vi "Text control 2 v6.0.vi"() -> ()   [LabVIEW 2016]
panel:
  in  "Tab Control":enum32{"Main", "Other parameters"}(tab)
  out "Line running":i32
  out "Total lines":i32
  out "Path":path=path "C:/users/rlp38/09Apr2009LTtesting/test2.txt"
  out "I vs Vg":cluster{"Y data in":dbl[], "X data in":dbl[]}[](graph)
  out "Is max":dbl format="%.2e"
  out "Id max":dbl format="%.2e"
  out "Ig max":dbl format="%.2e"
  out "Imax vs time":cluster{"Y data in":dbl[], "X data in":dbl[]}[](graph)
  out "Imin vs time":cluster{"Y data in":dbl[], "X data in":dbl[]}[](graph)
  out "I vs Vd":cluster{"Y data in":dbl[], "X data in":dbl[]}[](graph)
  in  "Script":string="#pulsedstressV d 0.03 20 0 0.5 0.0827 5\n#\n#itime m\n#gaterangemode a\n#drainrangemode a\n#pulsed on 0.05 0 0.02\n#transfer d -10 40 1 5 40 35\n#transfer d -10 40 1 5 40 35\n#transfer d -10 40 1 5 40 35\n#output d 0 40 20 0 40 1\n#\n#\n#sample 1 0.008 221 6 0.003\n#samplei 400e-6 200 6 0.002 0.1\n#vsu2pulse -10 4\n#\n#stressV 0.016 0.03 2e-4 0.1e-3 11\n#stressI 220e-7 0.08 15\n#transfer s -1 1 0.5 -0.005 0.005 0.005\n#output s 0 0 0 -0.008 0.008 0.002"
  out "Command running:":string
  out "Serial port data":string
  out "Elapsed Time":dbl caption="Elapsed Time (s)"
  in  "Units (label only)":u16(ring)=1 items=["Seconds", "Minutes", "Hours"]
  in  "Time Offset":dbl caption="Set Start Time (s)"
  in  "Reset":bool
  in  "Auto Reset":bool
  in  "integration time":u32(slide) max=2 step=1 scale=0.0..2.0
  out "Is on":dbl format="%.2e"
  out "Id on":dbl format="%.2e"
  out "Ig on":dbl format="%.2e"
  out "Ion vs time":cluster{"Y data in":dbl[], "X data in":dbl[]}[](graph)
  out "Ioff vs time":cluster{"Y data in":dbl[], "X data in":dbl[]}[](graph)
  out "Ig min":dbl format="%.2e"
  out "Id min":dbl format="%.2e"
  out "Is min":dbl format="%.2e"
  out "Is off":dbl format="%.2e"
  out "Id off":dbl format="%.2e"
  out "Ig off":dbl format="%.2e"
  in  "Integration time (long)":dbl=0.32 min=0.04 max=2.0 step=0.02 format="%.2f"
  in  "Integration time (short)":dbl=0.0019 min=8e-05 max=0.0019 step=8e-05 format="%^.0e"
  in  "Drain: Compliance":dbl=0.001 format="%.8f"
  in  "Gate: Compliance":dbl=0.001 format="%.8f"
  in  "Interrupt run":bool
  in  "Standby":T1
  in  "Full Reset":bool
  in  "SMU4":cluster{"on/off":bool, "Voltage":dbl} {"Voltage" min=-100.0 max=100.0 format="%.2f"}
  in  "Gate Range\nmode":u16(ring) items=["Auto", "Limited", "Fixed"]
  in  "Gate Range":u8(slide)=6 max=11 scale=0.0..11.0
  in  "Source/Drain\nRange mode":u16(ring) items=["Auto", "Limited", "Fixed"]
  in  "Source/Drain Range":u8(slide)=6 max=11 scale=0.0..11.0
  in  "Panel Controls":T2={"Emergency Stop"=refnum, "TransGraph Max"=1e-05, "Text/Graph (text=false)"=TRUE} {"TransGraph Max" format="%.2e"}
  in  "Panel Controls 2":T3={"Emergency Stop"=refnum, "TransGraph Max"=1e-05, "Text/Graph (text=false)"=TRUE, "TransGraph Min"=1e-11} {"TransGraph Min" format="%.2e"; "TransGraph Max" format="%.2e"}
  out "error out":errorcluster
  in  "Delay before read (ms)":u32=1000
  in  "byte count":u32=64
  in  "Serial End Mode for Reads":u16(ring)=2 items=["None", "LastBit", "TermChar"]
  in  "Timeout (ms)":u32=10000
  in  "Enable Termination\nChar (T)":bool=TRUE
  in  "Termination char\n(0xA = '\\n' = LF)\n(0xD = '\\r' = CR)":u8=13 format="%.0x"
  in  "flow control":u16(ring) items=["None"=0, "XON/XOFF"=1, "RTS/CTS"=2, "DTR/DSR"=4]
  in  "stop bits":u16(ring)=10 items=["1.0"=10, "1.5"=15, "2.0"=20]
  in  "parity":u16(ring) items=["None", "Odd", "Even", "Mark", "Space"]
  in  "data bits":u16=8 min=5 max=8 step=1
  in  "VISA resource name":refnum<visa-resource-name>="COM6"
  in  "baud rate":u32=9600
  out "Timings Indicator":T4
  in  "Timings (overwritten by the Front Panel)":T5={"integration time"=0, "Short/Long integration time"=0.00064, "hold time (sec)"=0.0, "delay time (sec)"=0.0, "Step Time (0 disables)"=0.0, "sweep method"=0, "Pulse period"=0.005, "Base voltage"=0.0, "Pulse width"=0.0005} {"Pulse width" min=0.0005 max=0.1 step=0.0001 format="%.4f"; "Base voltage" format="%^.4e"; "Pulse period" min=0.005 max=1.0 step=0.0001 format="%.4f"; "sweep method" items=["Continuous", "Pulsed"]; "Step Time (0 disables)" format="%.2f"; "delay time (sec)" format="%.4f"; "hold time (sec)" format="%.4f"; "Short/Long integration time" format="%^.0e"; "integration time" scale=0.0..2.0}
  in  "Gate":T6={"Gate Start"=0.0, "Gate Stop"=2.0, "Gate Step (linear only)"=1.0, "Gate Compliance"=0.0001, "Gate PComp"=0.0, "Range mode"=0, "Range"=6} {"Range" max=11 scale=0.0..11.0; "Range mode" items=["Auto", "Limited", "Fixed"]; "Gate PComp" format="%^.2e"; "Gate Compliance" format="%^.2e"; "Gate Step (linear only)" format="%^.4e"; "Gate Stop" format="%^.4e"; "Gate Start" format="%^.4e"}
  in  "Drain 2":T7={"Drain Start"=0.0, "Drain Stop"=2.0, "Drain Compliance"=0.0001, "Drain Step"=1.0, "Drain PComp"=0.0, "Range mode"=0, "Range"=6} {"Range" max=11 scale=0.0..11.0; "Range mode" items=["Auto", "Limited", "Fixed"]; "Drain PComp" format="%^.2e"; "Drain Step" format="%^.4e"; "Drain Compliance" format="%^.2e"; "Drain Stop" format="%^.4e"; "Drain Start" format="%^.4e"}
  # "Time"
  # "Syntax:\nitime [s|m|l] time(sec): [s|m|l] determines the integration time setting (small|medium|long) and time sets the value.\nNOTE: The value of the integration time has to be within the range allowed by its category (s|m|l), otherwise, the closest value will be used. (e.g. if the category is set to short but the time value is very long, the actual value used will be the maximum short integration time.\nIntegration times:\n    Short: Default: 640 us. Range: 8E-5 - 1.92E-3 seconds.\n    Medium: Fixed at 1 NPL cycle (0.02 seconds).\n    Long: Default: 16 NPL cycles (0.32 seconds). Range: 2-100 NPL cycles (0.04 seconds - 2 seconds).\ngaterangemode [a|l|f]\ndrainrangemode [a|l|f]\npulsed [on|off] PulsePeriod(sec) PulseBaseVoltage PulseONWidth(sec)\nstandby [on l off]\nwait NumMilliseconds\nwait-min NumMinutes\n# texthere = comment\ntransfer [s|d] VgStart VgStop VgStep VdStart VdStop VdStep\noutput [s|d] VgStart VgStop VgStep VdStart VdStop VdStep\nsample Vg Vd NumSamples Time(s) SampleInterval(s)\nsamplei Idg NumSamples Time(s) SampleInterval(s) VDGcompliance\n100 samples is approximately 13 seconds with medium integration\n# if in doubt use SampleInterval(s) = 0.004\nstressV VG VD IGcompliance IDcompliance Duration(sec)\nstressI IDG VDGcompliance Duration(sec)\nvsu2pulse Bias Duration(s)\npulsedstressV [s|d] VEstop VgON VgOFF Period(s) PulseONwidth(s) Vd\nsample-fpp Vg Vd NumSamples Time\nresample-fpp Vg Vd\ntransfer-fpp [s|d] VgStart VgStop VgStep VdStart VdStop VdStep\noutput-fpp [s|d] VgStart VgStop VgStep VdStart VdStop VdStep\nserial SerialPortCommand"
  # "1\n2\n3\n4\n5\n6\n7\n8\n9\n10\n11\n12\n13\n14\n15\n16\n17\n18\n19\n20"
  # "Serial port settings"
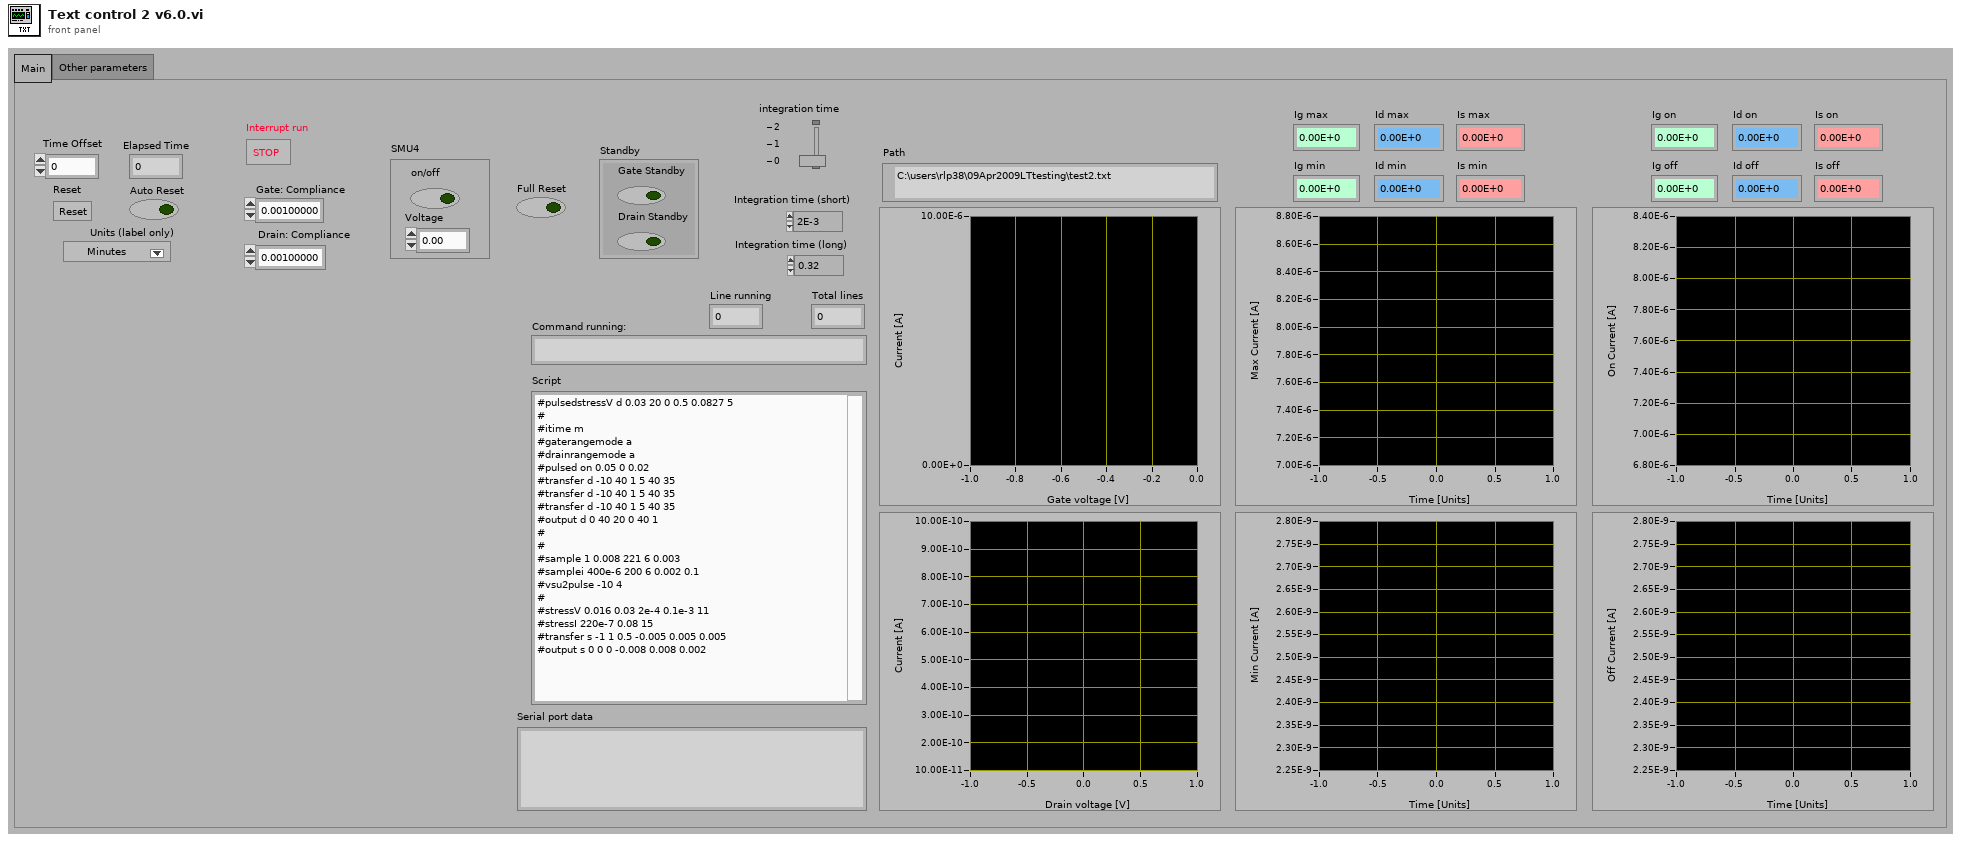
[diagram p1: front panel]
types:
  T1 = cluster{"Gate Standby":bool, "Drain Standby":bool}
  T2 = cluster{"Emergency Stop":refnum<vi>, "TransGraph Max":dbl, "Text/Graph (text=false)":bool}
  T3 = cluster{"Emergency Stop":refnum<vi>, "TransGraph Max":dbl, "Text/Graph (text=false)":bool, "TransGraph Min":dbl}
  T4 = cluster{"integration time (0:s, 1:m, 2:l)":u32, "Short/Long integration time":dbl, "hold time (sec)":dbl, "delay time (sec)":dbl, "Step Time (0 disables)":dbl, "sweep method":u16, "Pulse period":dbl, "Base voltage":dbl, "Pulse width":dbl}
  T5 = cluster{"integration time":u32, "Short/Long integration time":dbl, "hold time (sec)":dbl, "delay time (sec)":dbl, "Step Time (0 disables)":dbl, "sweep method":u16, "Pulse period":dbl, "Base voltage":dbl, "Pulse width":dbl}
  T6 = cluster{"Gate Start":dbl, "Gate Stop":dbl, "Gate Step (linear only)":dbl, "Gate Compliance":dbl, "Gate PComp":dbl, "Range mode":u16, "Range":u8}
  T7 = cluster{"Drain Start":dbl, "Drain Stop":dbl, "Drain Compliance":dbl, "Drain Step":dbl, "Drain PComp":dbl, "Range mode":u16, "Range":u8}
  T8 = enum16{"open", "replace", "create", "open or create", "replace or create", "replace or create with confirmation"}
  T9 = cluster{"V2 Start":dbl, "V2 Step":dbl, "Number of points":i32}
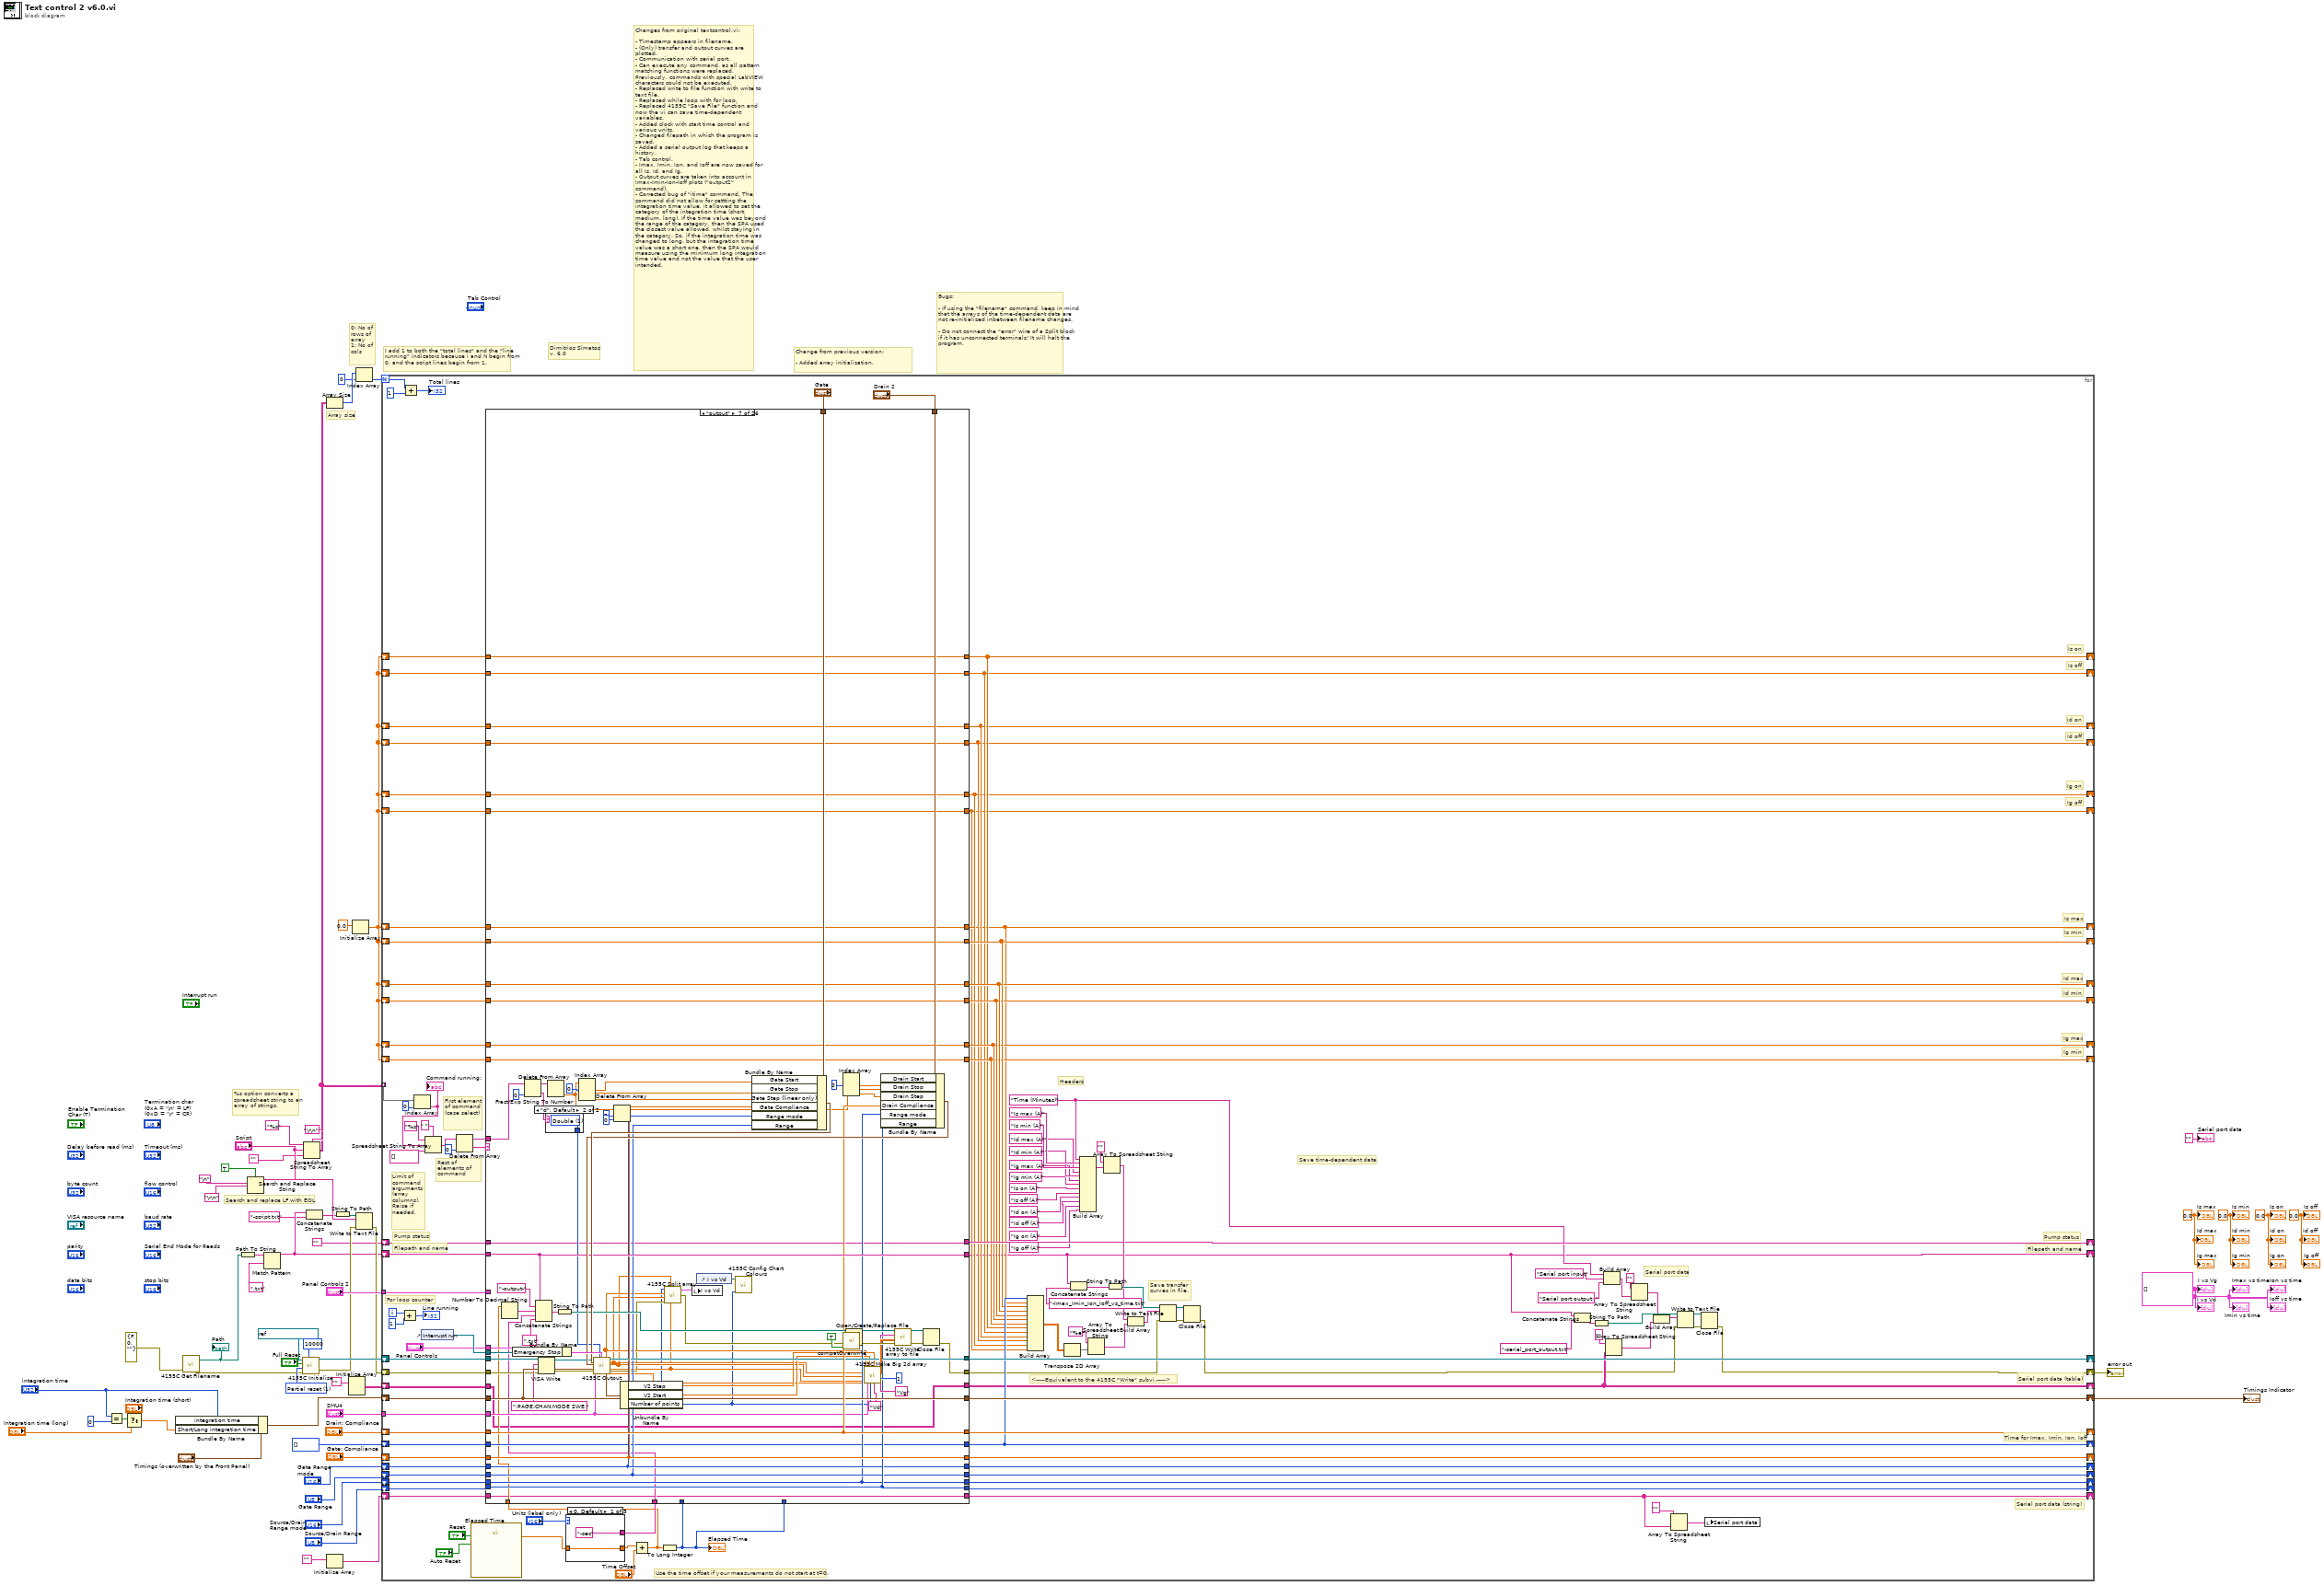
[diagram p0: block diagram]
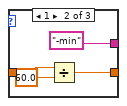
[diagram p2: hidden frame]
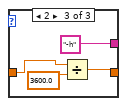
[diagram p3: hidden frame]
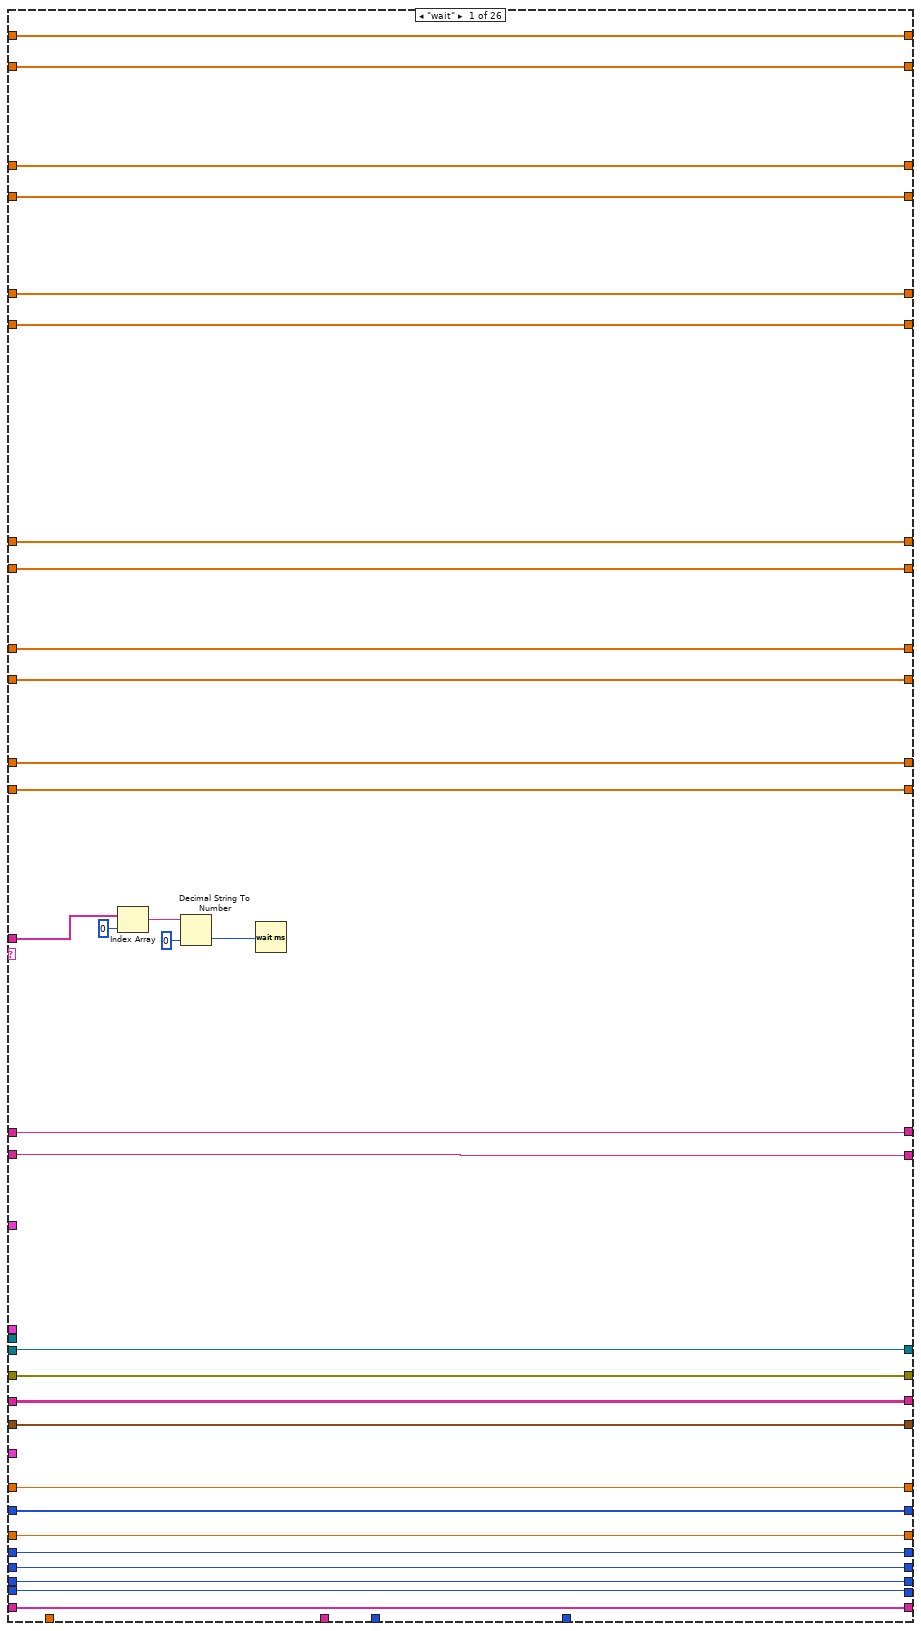
[diagram p4: hidden frame]
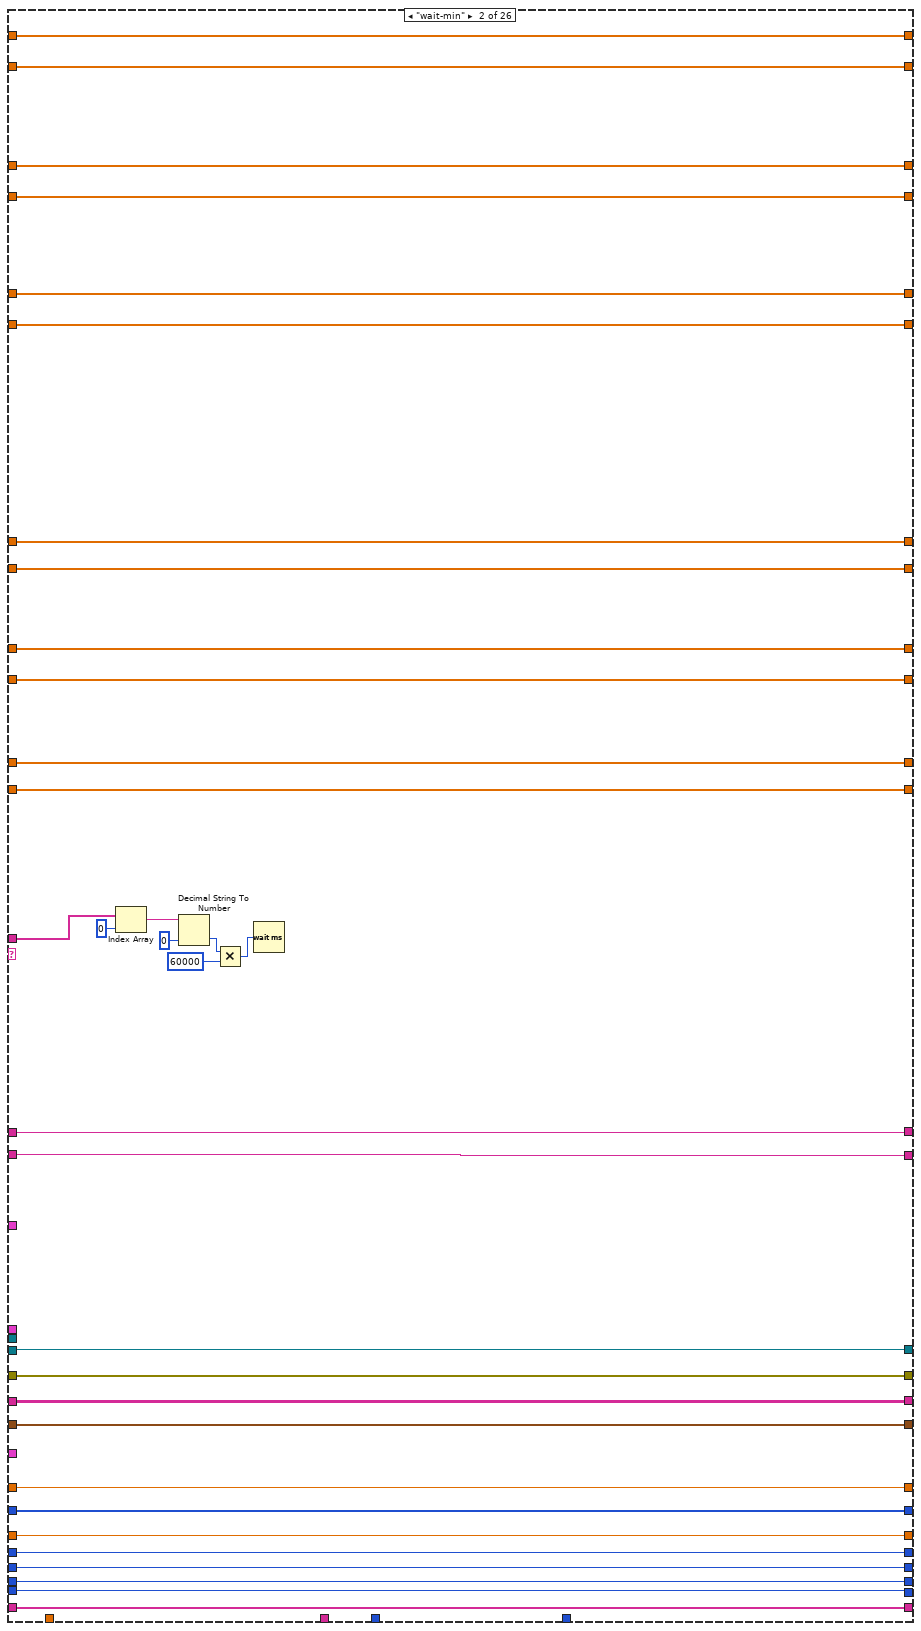
[diagram p5: hidden frame]
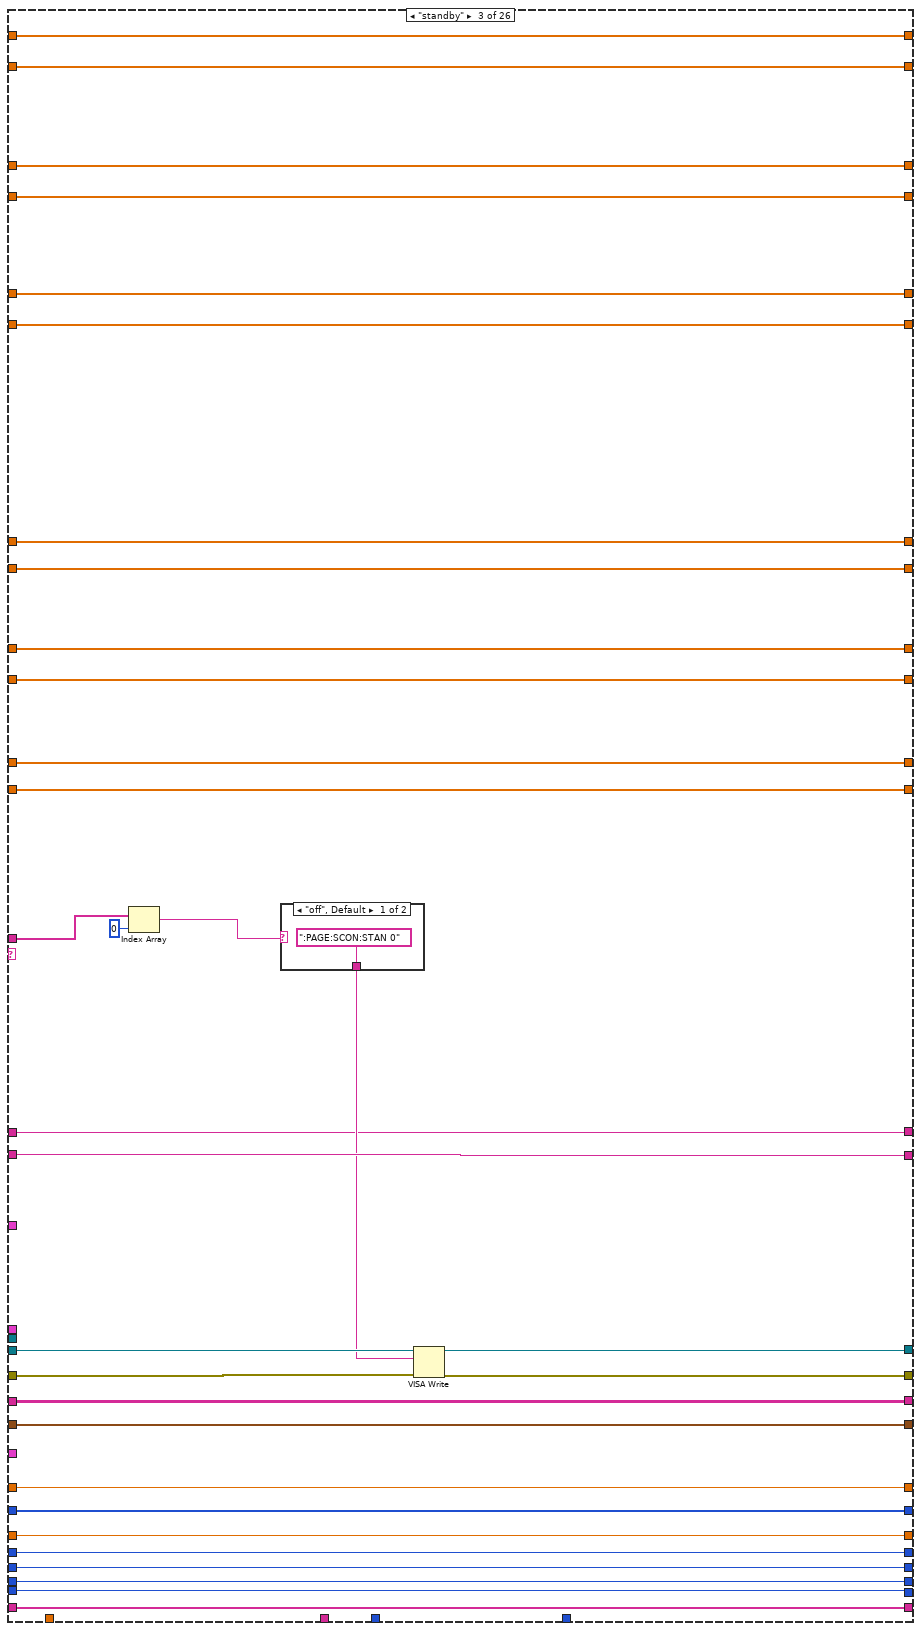
[diagram p6: hidden frame]
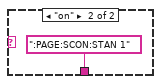
[diagram p7: hidden frame]
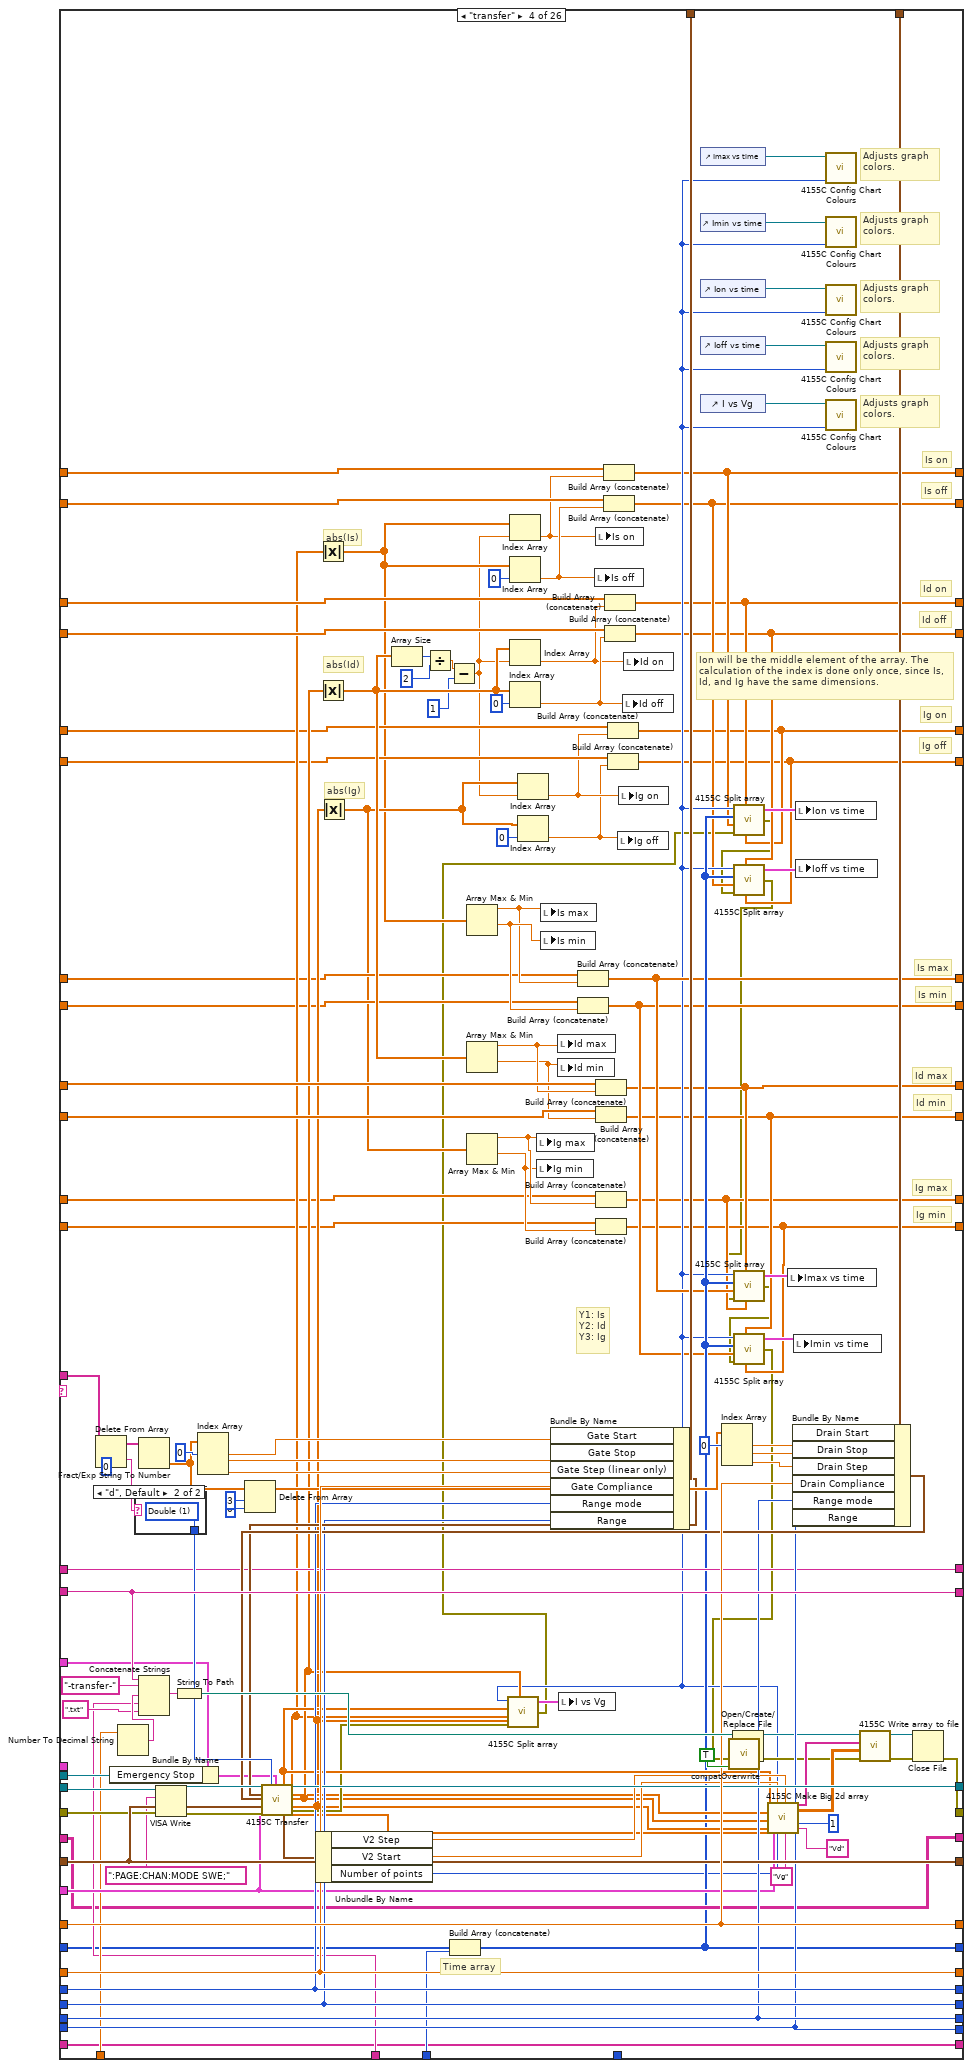
[diagram p8: hidden frame]
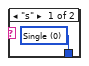
[diagram p9: hidden frame]
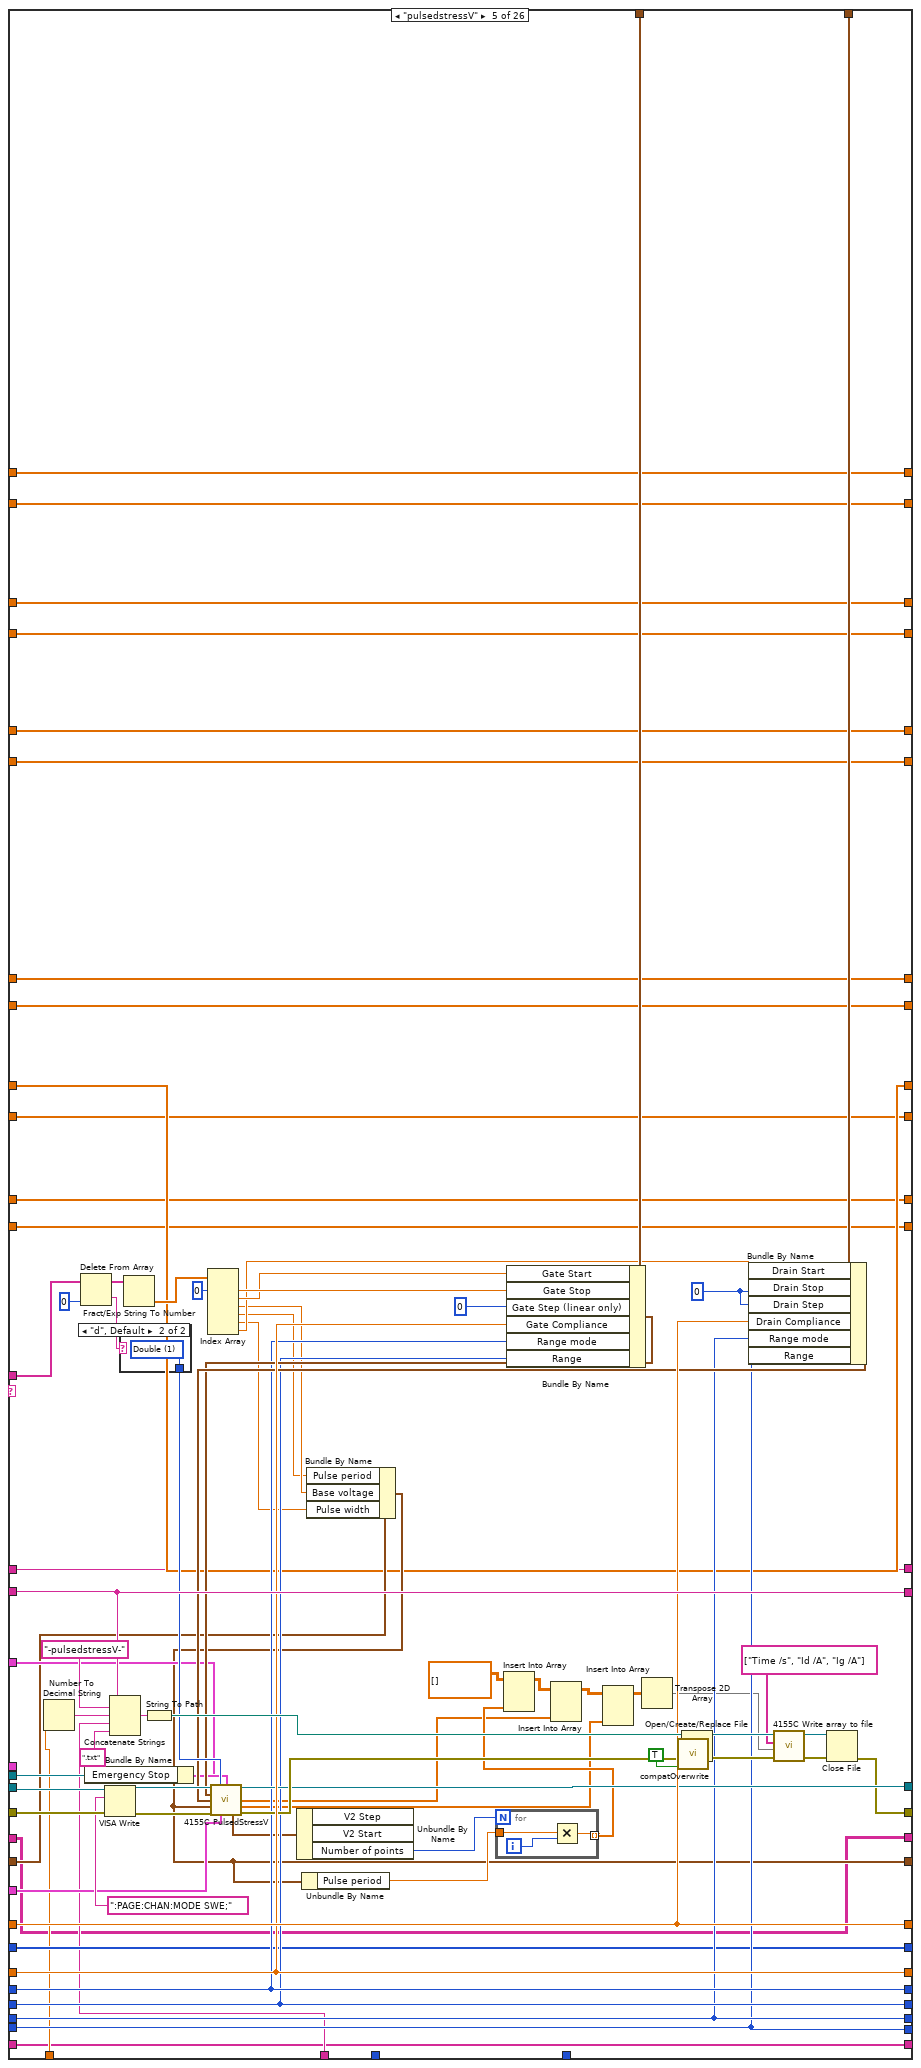
[diagram p10: hidden frame]
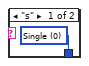
[diagram p11: hidden frame]
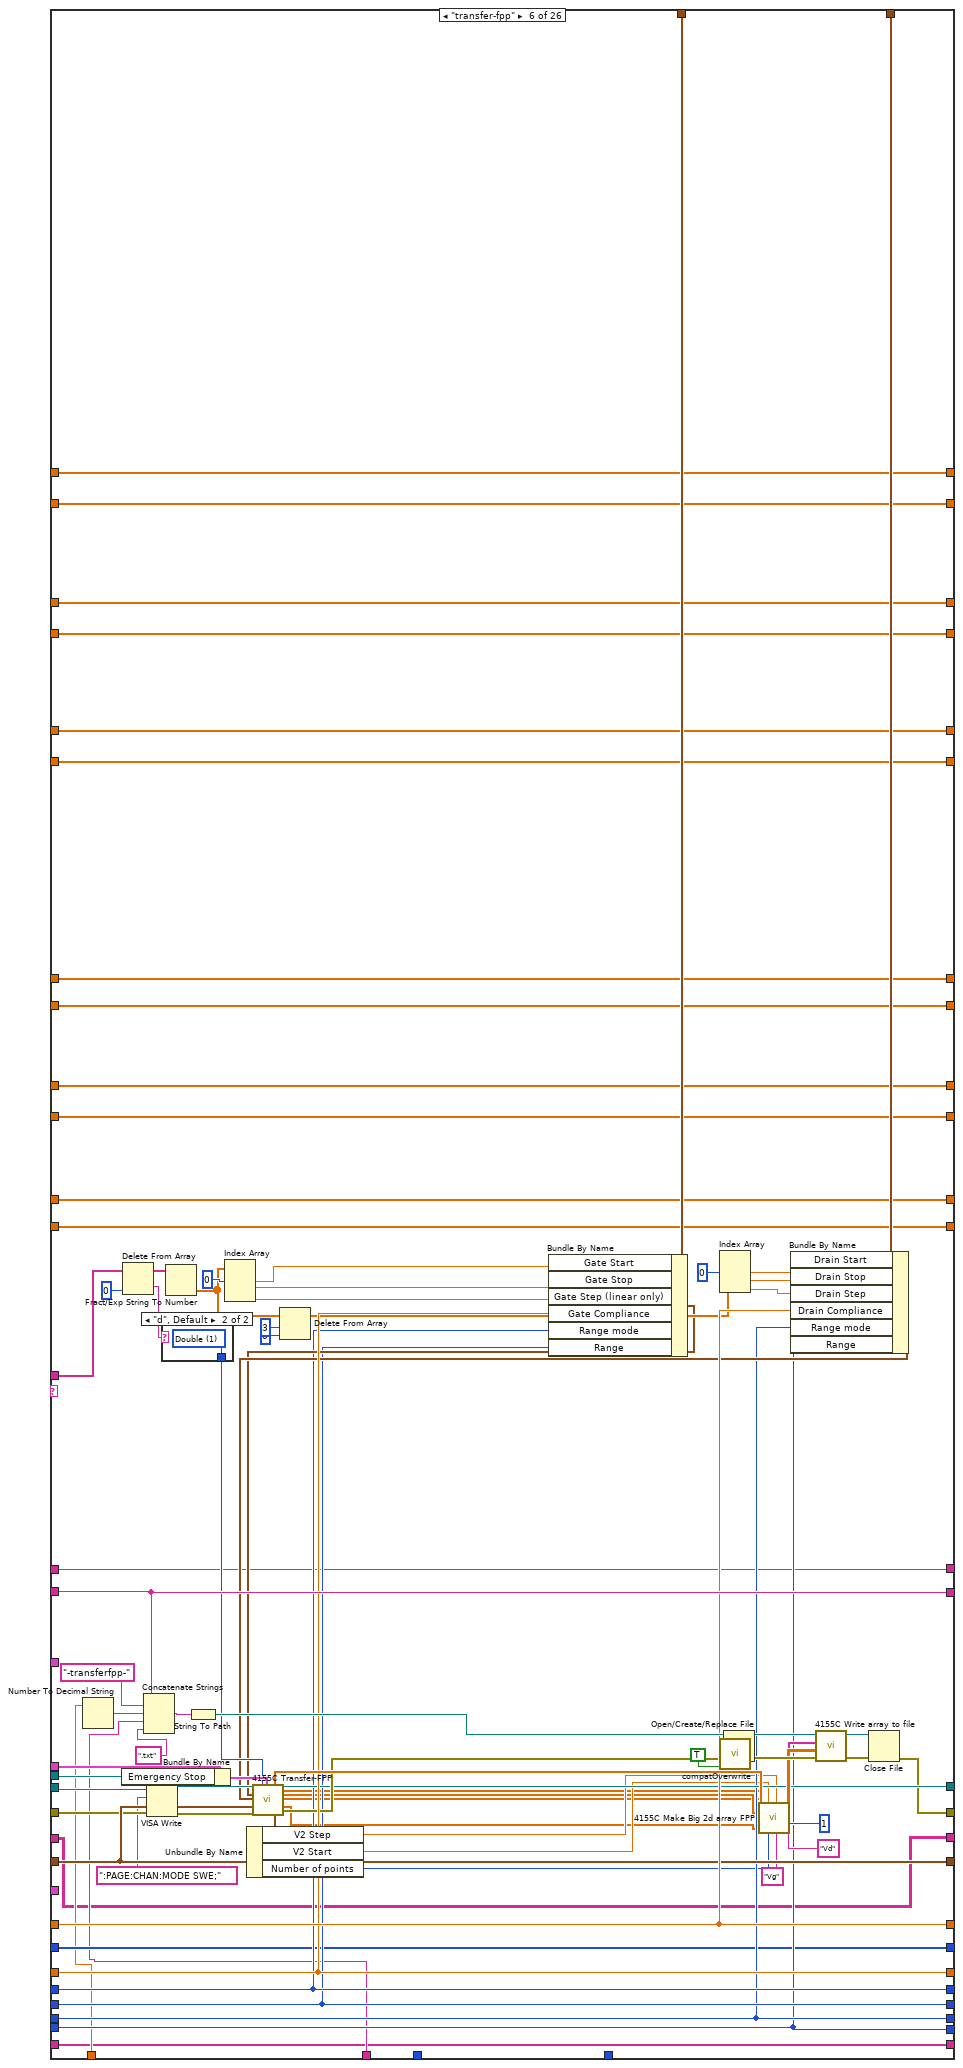
[diagram p12: hidden frame]
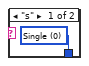
[diagram p13: hidden frame]
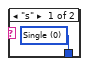
[diagram p14: hidden frame]
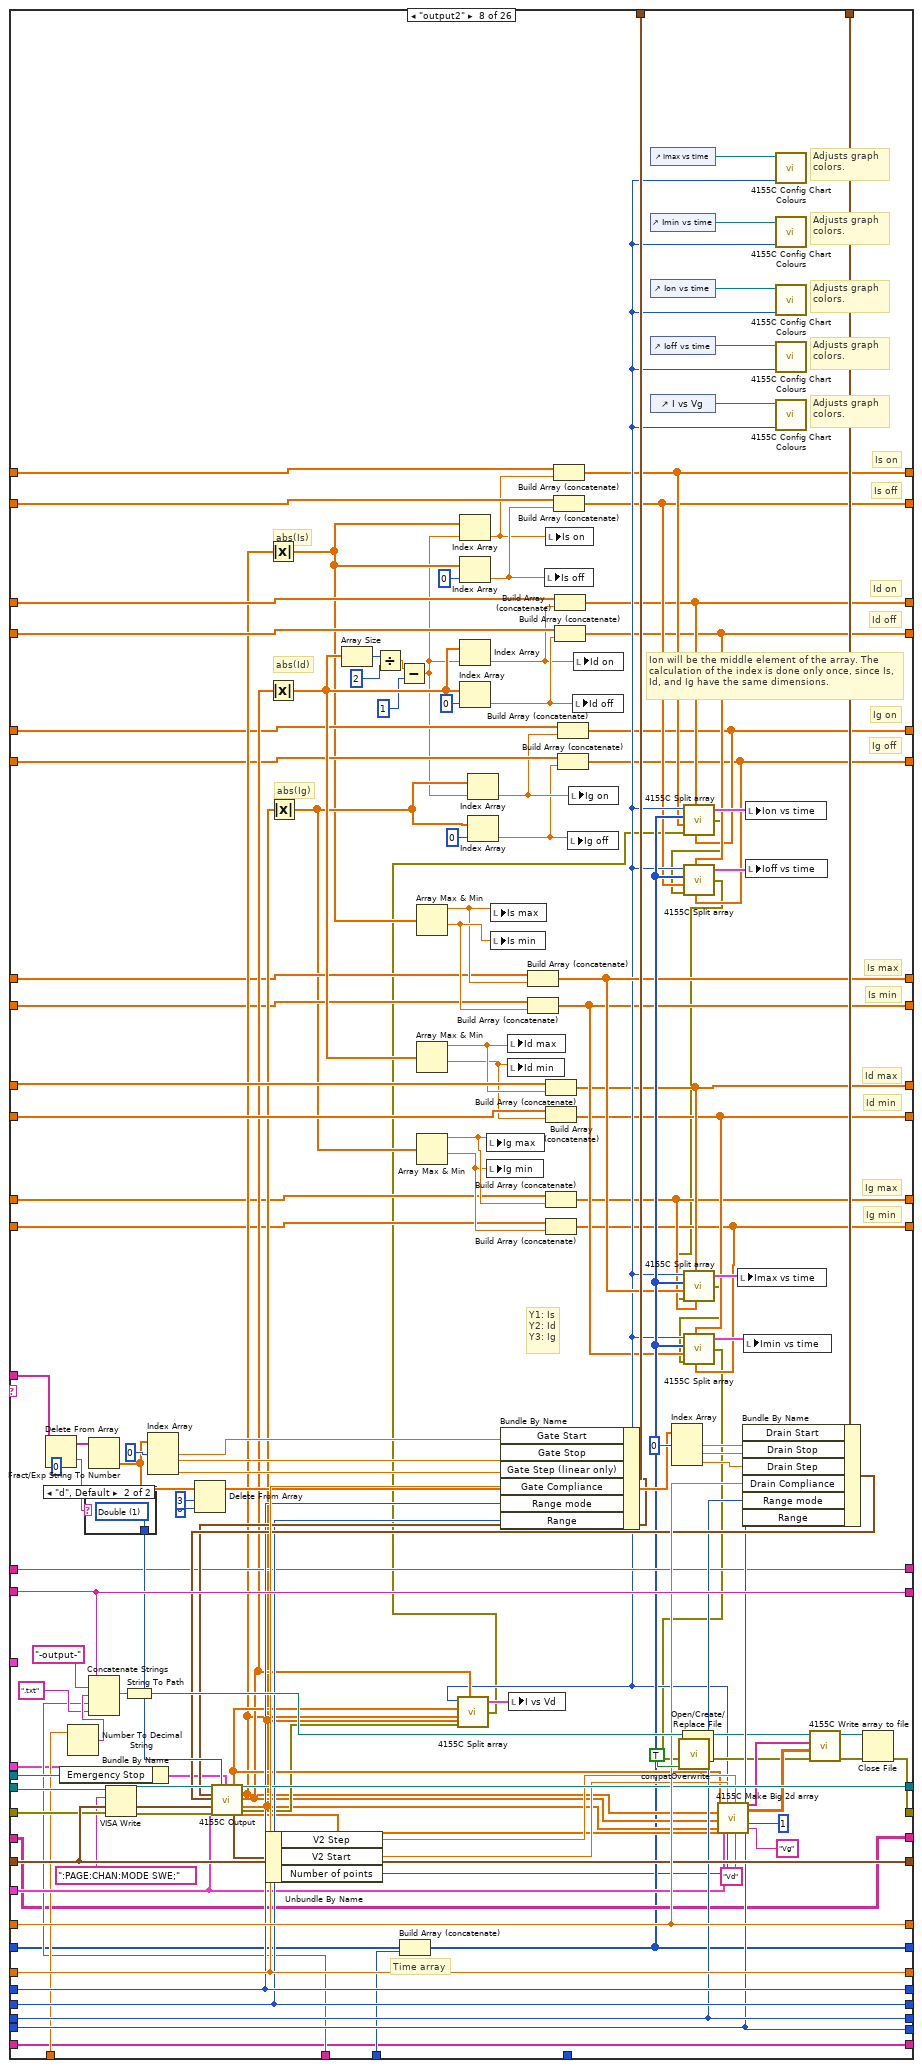
[diagram p15: hidden frame]
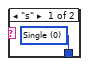
[diagram p16: hidden frame]
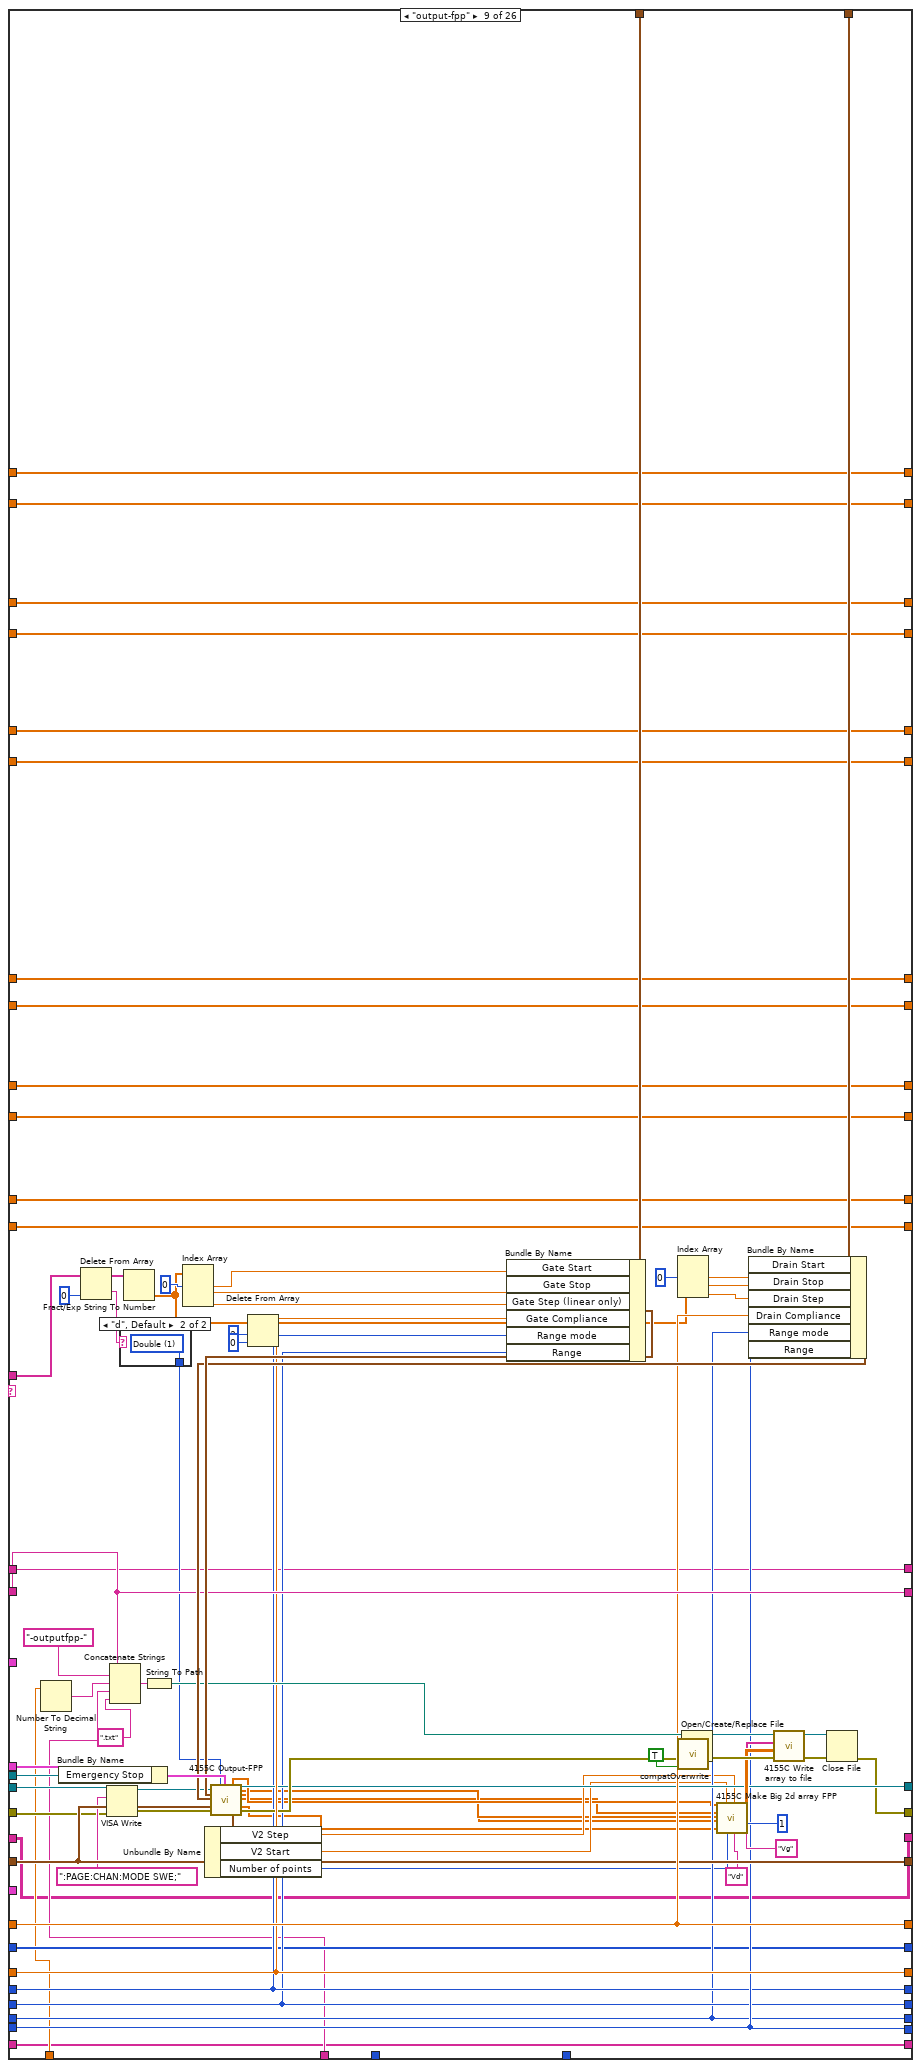
[diagram p17: hidden frame]
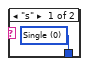
[diagram p18: hidden frame]
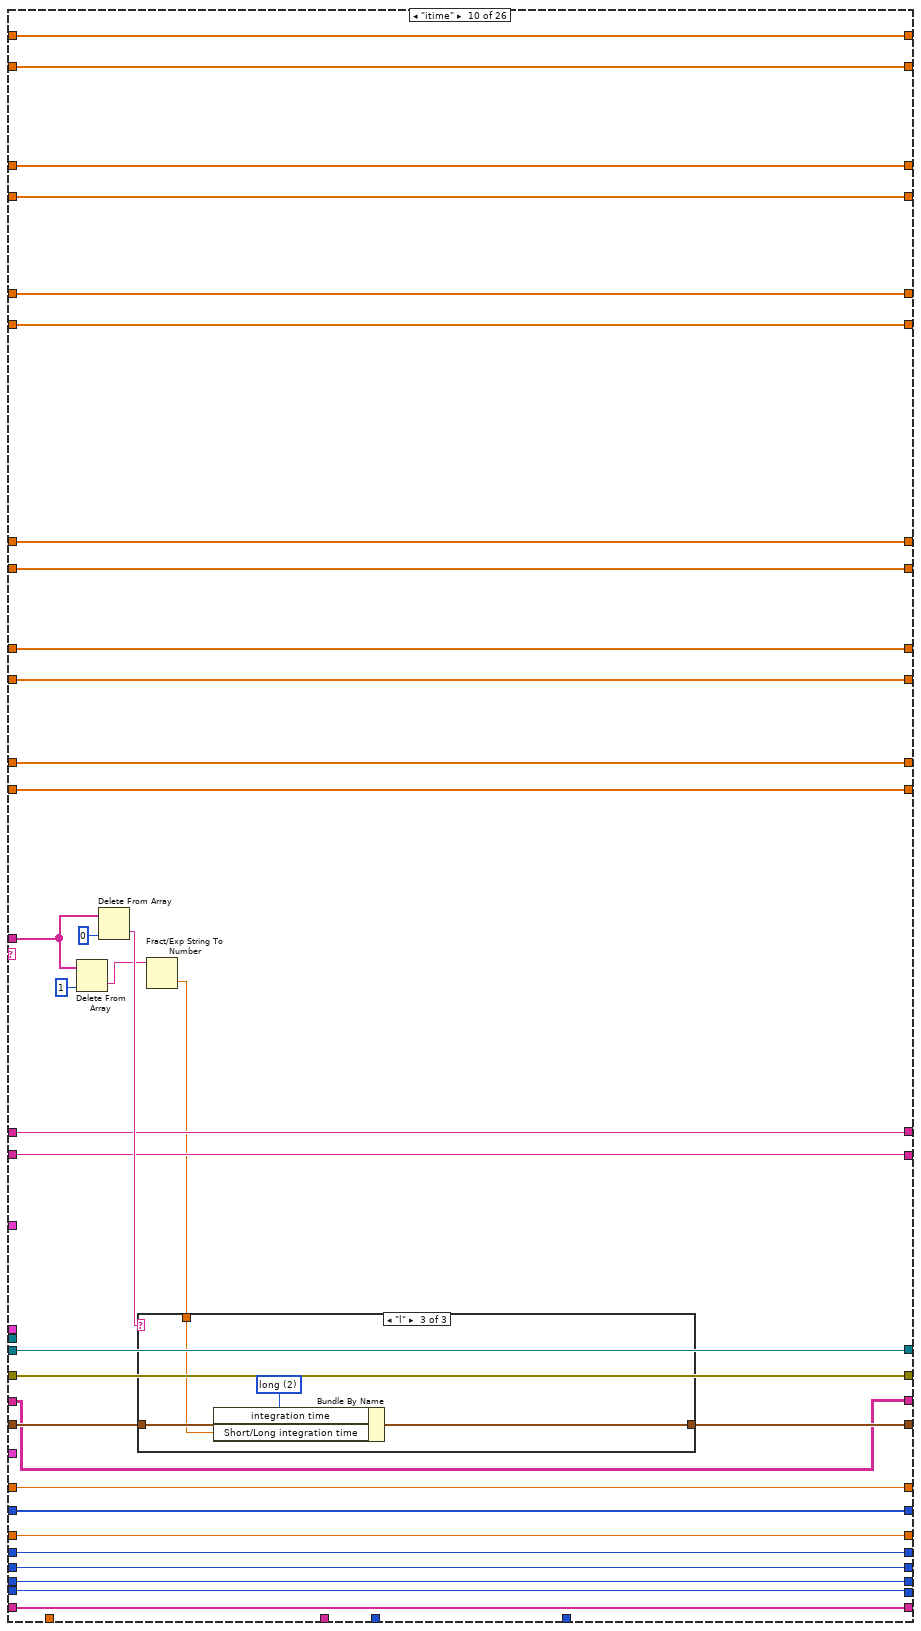
[diagram p19: hidden frame]
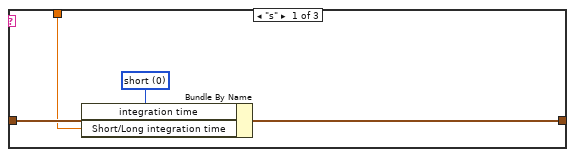
[diagram p20: hidden frame]
diagram:
  w2 = cluster{"Y data in":dbl[], "X data in":dbl[]}[] [] ("I vs Vg")
  w3 = 0.0 ("Is off")
  w4 = 0.0 ("Is on")
  w5 = 0.0 ("Is min")
  w6 = 0.0 ("Is max")
  w55 = u16 1 items=["Reset All", "Partial reset"] ("Type of reset")
  # "Change from previous version:\n\n- Added array initialization."
  # "I add 1 to both the \"total lines\" and the \"line running\" indicators because i and N begin from 0, and the script lines begin from 1."
  # "Bugs:\n\n- If using the \"filename\" command, keep in mind that the arrays of the time-dependent data are not re-initialized inbetween filename changes. \n\n- Do not connect the \"error\" wire of a Split block if it has unconnected terminals! It will halt the program."
  # "Array size"
  # "%s option converts a spreadsheet string to an array of strings."
  # "0: No of rows of array\n1: No of cols"
  # "Dimitrios Simatos\nv. 6.0"
  # "Changes from original textcontrol.vi:\n\n- Timestamp appears in filename.\n- (Only) transfer and output curves are plotted.\n- Communication with serial port.\n- Can execute any command, as all pattern matching functions were replaced. Previously, commands with special LabVIEW characters could not be executed.\n- Replaced write to file function with write to text file.\n- Replaced while loop with for loop.\n- Replaced 4155C \"Save File\" function and now the vi can save time-dependent variables.\n- Added clock with start time control and various units.\n- Changed filepath in which the program is saved.\n- Added a serial output log that keeps a history.\n- Tab control.\n- Imax, Imin, Ion, and Ioff are now saved for all Is, Id, and Ig.\n- Output curves are taken into account in Imax-Imin-Ion-Ioff plots (\"output2\" command).\n- Corrected bug of \"itime\" command. The command did not allow for settting the integration time value, it allowed to set the category of the integration time (short, medium, long). If the time value was beyond the range of the category, then the SPA used the closest value allowed, whilst staying in the category. So, if the integration time was changed to long, but the integration time value was a short one, then the SPA would measure using the minimum long integration time value and not the value that the user intended."
  # "Search and replace LF with EOL"
  n1 = Equal?(x="integration time", y=u32 0) -> (x = y?=w56:bool)
  n2 = Select(t="Integration time (short)", s=w56, f="Integration time (long)") -> (s? t:f=w11:dbl)
  n3 = Bundle By Name(cluster="Timings (overwritten by the Front Panel)", "integration time"="integration time", "Short/Long integration time"=w11) -> (w48:T5)
  n4 = call "4155C Get Filename.vi"("error in (no error)"=errorcluster {"status"=FALSE, "code"=0, "source"=""}) -> ("error out"=w50:errorcluster, "path"=w25:path)  [unwired: 2 in, 1 out]
  "Path" <- w25
  n5 = Path To String(path=w25) -> (string=w26:string)
  n6 = Search and Replace String(replace all?=TRUE ("replace all? (F)"), input string="Script", search string="\n", replace string="\r\n") -> (result string=w38:string)  [unwired: 4 in, 3 out]
  n7 = Match Pattern(string=w26, regular expression=".txt") -> (before substring=w9:string)  [unwired: 1 in, 3 out]
  n8 = call "4155C Initialise.vi"("VISA resource name in"=refnum<visa-resource-name> "GPIB0::14::INSTR", "Reset"="Full Reset", "Type of reset"=w55, "error in (no error)"=w50, "VISA Timeout Value"=u32 10000) -> ("VISA Resource Name out"=w49:refnum<visa-resource-name>, "error out"=w21:errorcluster)
  n9 = Spreadsheet String To Array(delimiter (Tab)="\r\n", format string="%s", spreadsheet string="Script", array type (2D Dbl)="") -> (array=w29:string[][])
  n10 = Concatenate Strings(w9, "-script.txt" ("string")) -> (w10:string)
  n11 = Array Size(array=w29) -> (size(s)=w33:i32[])
  n12 = Initialize Array("") -> (w16:string[])  [unwired: 1 in]
  n13 = String To Path(string=w10) -> (path=w22:path)
  n14 = Initialize Array("") -> (w14:string[][])  [unwired: 2 in]
  n15 = Initialize Array(0.0 ("element")) -> (w18:dbl[])  [unwired: 1 in]
  n16 = Index Array(array=w33, index=0) -> (element=w31:i32)
  n17 = Write to Text File(file (use dialog)=w22, text=w38, error in=w21) -> (error out=w20:errorcluster)  [unwired: 1 in, 2 out]
  n18 = for {
    N: w31 -> [w128]
    tunnel: "SMU4" -> [w164]
    shift-left: "Source/Drain Range" -> [w169]
    shift-right: [w165] -> _
    shift-left: "Source/Drain\nRange mode" -> [w170]
    shift-right: [w166] -> _
    shift-left: "Gate Range" -> [w171]
    shift-right: [w167] -> _
    shift-left: "Gate Range\nmode" -> [w172]
    shift-right: [w168] -> _
    shift-left: "Gate: Compliance" -> [w181]
    shift-right: [w177] -> _
    shift-left: "Drain: Compliance" -> [w182]
    shift-right: [w178] -> _
    shift-left: w48 -> [w183]
    shift-right: [w179] -> w12
    shift-left: w20 -> [w184]
    shift-right: [w62] -> w24
    shift-left: w49 -> [w185]
    shift-right: [w180] -> _
    shift-left: w9 -> [w186]
    shift-right: [w65] -> _
    tunnel: "Panel Controls 2" -> [w163]
    shift-right: [w77] -> _
    shift-left: w18 -> [w162]
    shift-right: [w113] -> _
    shift-left: i32[] [] -> [w158]
    tunnel: w29 -> [w157] mode=indexing
    shift-right: [w76] -> _
    shift-left: w18 -> [w134]
    shift-right: [w107] -> _
    shift-left: w16 -> [w120]
    shift-right: [w115] -> _
    shift-left: "" -> [w114]
    shift-right: [w108] -> _
    shift-left: w14 -> [w110]
    shift-right: [w70] -> _
    shift-left: w18 -> [w98]
    shift-right: [w71] -> _
    shift-left: w18 -> [w97]
    shift-right: [w75] -> _
    shift-left: w18 -> [w86]
    shift-right: [w74] -> _
    shift-left: w18 -> [w85]
    shift-right: [w68] -> _
    shift-left: w18 -> [w84]
    shift-right: [w78] -> _
    shift-left: w18 -> [w83]
    shift-right: [w69] -> _
    shift-left: w18 -> [w82]
    shift-right: [w67] -> _
    shift-left: w18 -> [w81]
    shift-right: [w73] -> _
    shift-left: w18 -> [w80]
    shift-right: [w72] -> _
    shift-left: w18 -> [w79]
    i -> [w123]
    w100 = "Time (Minutes)" ("element")
    # "Is off"
    # "Is on"
    # "Ig off"
    # "Ig on"
    # "Is min"
    # "Is max"
    # "Ig min"
    # "Ig max"
    # "Id min"
    # "Id max"
    # "Id off"
    # "Id on"
    # "Pump status"
    # "Filepath and name"
    # "Pump status"
    # "Limit of command arguments (array columns). Raise if needed."
    # "Serial port data (string)"
    # "Serial port data (table)"
    # "Serial port data"
    # "For loop counter"
    # "<-----Equivalent to the 4155C \"Write\" subvi.----->"
    # "Headers"
    # "Save transfer curves in file."
    # "Filepath and name"
    # "Save time-dependent data."
    # "Use the time offset if your measurements do not start at t=0."
    # "Time for Imax, Imin, Ion, Ioff"
    # "Rest of elements of command"
    # "First element of command\n(case select)"
    n19 = Add(x=w123, y=1) -> (x+y=→"Line running":i32)
    n20 = Add(x=w128, y=1) -> (x+y=→"Total lines":i32)
    n21 = Index Array(array=w157, index=0 ("line index")) -> (element=w152:string)
    "Command running:" <- w152
    n22 = control-ref of="Interrupt run"() -> (w176:refnum<vi>)
    n23 = Spreadsheet String To Array(delimiter (Tab)=" ", format string="%s", spreadsheet string=w152, array type (2D Dbl)=string[] []) -> (array=w150:string[])
    n24 = Delete From Array(array=w150, index=0) -> (deleted portion=w99:string, array with subset deleted=w149:string[])  [unwired: 1 in]
    n25 = call "Elapsed Time"("Reset"="Reset", "Auto Reset"="Auto Reset") -> ("Elapsed Time (s)"=w159:dbl)  [unwired: 10 in, 7 out]
    n26 = case shown="0, Default" "Units (label only)" {
      tunnel: ["-sec" "-min" "-h"] -> w160
      tunnel: [w187 w191 w194] -> w130
      tunnel: w159 -> [w187 w190 w195]
      frame 0, Default {
      }
      frame 1 {
        n27 = Divide(x=w190, y=60.0) -> (x/y=w191:dbl)
      }
      frame 2 {
        n28 = Divide(x=w195, y=3600.0) -> (x/y=w194:dbl)
      }
    }
    n29 = Add(x=w130, y="Time Offset") -> (x+y=w129:dbl)
    n30 = To Long Integer(number=w129) -> (32bit integer=w112:i32)
    "Elapsed Time" <- w112
    n31 = case shown="\"output\"" w99 {
      tunnel: w149 -> [w227 w260 w292 w420 w443 w580 w670 w818 w891 w918 w988 w1029 w1068 w1103 w1131 _ _ w1277 w1352 _ w1445 w1503 w1559 w1643 w1719 w1753]
      tunnel: w186 -> [w222 w256 w290 w427 w504 w588 w677 w825 w899 w936 w977 w1021 w1061 w1097 w1124 w1157 w1213 w1255 w1334 w1379 w1432 w1490 w1547 w1637 w1715 w1755]
      tunnel: w185 -> [w221 w255 w281 w398 w489 w557 w646 w796 w867 w937 w978 w1022 w1062 w1098 w1125 w1162 w1215 w1283 w1358 w1383 w1451 w1509 w1565 w1649 w1673 w1759]
      tunnel: w184 -> [w220 w254 w280 w397 w488 w556 w643 w795 w864 w938 w979 w1023 w1063 w1099 w1126 w1161 w1186 w1282 w1357 w1382 w1450 w1508 w1564 w1648 w1672 w1758]
      tunnel: w183 -> [w219 w253 w289 w423 w464 w584 w673 w821 w895 w946 w987 w1020 w1060 w1096 w1123 w1160 w1210 w1246 w1326 w1388 w1425 w1483 w1540 w1636 w1714 w1760]
      tunnel: w182 -> [w218 w252 w288 w425 w502 w586 w675 w823 w897 w945 w986 w1028 w1067 w1102 w1130 w1159 w1195 w1281 w1356 w1391 w1449 w1507 w1563 w1647 w1723 w1761]
      tunnel: w181 -> [w217 w251 w287 w424 w501 w585 w674 w822 w896 w944 w985 w1027 w1066 w1101 w1129 w1158 w1196 w1256 w1335 w1390 w1433 w1491 w1548 w1638 w1716 w1763]
      tunnel: [w221 w255 w279 w422 w499 w582 w672 w820 w893 w937 w978 w1022 w1062 w1098 w1125 w1162 w1215 w1247 w1308 w1381 w1426 w1484 w1541 w1589 w1675 w1759] -> w180
      tunnel: [w220 w254 w278 w421 w498 w581 w671 w819 w892 w938 w979 w1023 w1063 w1099 w1126 w1161 w1185 w1257 w1309 w1380 w1434 w1492 w1549 w1588 w1674 w1757] -> w111
      tunnel: [w219 w253 w289 w423 w460 w584 w673 w821 w895 w939 w980 w1020 w1060 w1096 w1123 w1160 w1210 w1246 w1326 w1388 w1425 w1483 w1540 w1636 w1714 w1760] -> w179
      tunnel: [w218 w252 w288 w425 w502 w586 w675 w823 w897 w945 w986 w1028 w1067 w1102 w1130 w1159 w1195 w1281 w1356 w1391 w1449 w1507 w1563 w1647 w1723 w1761] -> w178
      tunnel: [w217 w251 w287 w424 w501 w585 w674 w822 w896 w944 w985 w1027 w1066 w1101 w1129 w1158 w1196 w1256 w1335 w1390 w1433 w1491 w1548 w1638 w1716 w1763] -> w177
      tunnel: [w222 w256 w290 w427 w504 w588 w677 w825 w899 w936 w977 w1021 w1061 w1097 w1124 w1157 w1213 w1255 w1334 w1379 w1432 w1490 w1547 w1637 w1715 w1755] -> w65
      tunnel: w176 -> [_ _ _ w429 w508 w593 w680 w827 w903 _ _ _ _ _ _ _ _ w1252 w1331 _ w1431 w1489 w1546 w1609 w1691 _]
      tunnel: "Gate" -> [_ _ _ w407 w492 w567 w657 w805 w878 _ _ _ _ _ _ _ _ _ _ _ _ _ _ _ _ _]
      tunnel: "Drain 2" -> [_ _ _ w406 w491 w566 w656 w804 w877 _ _ _ _ _ _ _ _ _ _ _ _ _ _ _ _ _]
      tunnel: "Panel Controls" -> [_ _ _ _ _ w565 w655 w694 w876 _ _ _ _ _ _ _ _ _ _ _ _ _ _ _ _ _]
      tunnel: w172 -> [w216 w250 w286 w391 w482 w550 w641 w789 w862 w943 w984 _ w1059 w1095 w1122 w1156 w1197 w1242 w1322 w1384 w1421 w1479 w1536 w1632 w1710 w1764]
      tunnel: w171 -> [w215 w249 w285 w390 w481 w549 w640 w788 w861 w942 w983 w1026 _ w1086 w1128 w1155 w1198 w1243 w1323 w1385 w1422 w1480 w1537 w1633 w1711 w1765]
      tunnel: w170 -> [w214 w248 w284 w389 w480 w548 w639 w787 w860 w941 w982 w1025 w1065 w1100 _ w1154 w1199 w1244 w1324 w1386 w1423 w1481 w1538 w1634 w1712 w1766]
      tunnel: w169 -> [w213 w247 w283 w388 w479 w547 w642 w786 w863 w940 w981 w1024 w1064 _ w1127 w1153 w1200 w1245 w1325 w1387 w1424 w1482 w1539 w1635 w1713 w1767]
      tunnel: [w216 w250 w286 w391 w482 w550 w641 w789 w862 w943 w984 w1019 w1059 w1095 w1122 w1156 w1197 w1242 w1322 w1384 w1421 w1479 w1536 w1632 w1710 w1764] -> w168
      tunnel: [w215 w249 w285 w390 w481 w549 w640 w788 w861 w942 w983 w1026 w1051 w1086 w1128 w1155 w1198 w1243 w1323 w1385 w1422 w1480 w1537 w1633 w1711 w1765] -> w167
      tunnel: [w214 w248 w284 w389 w480 w548 w639 w787 w860 w941 w982 w1025 w1065 w1100 w1121 w1154 w1199 w1244 w1324 w1386 w1423 w1481 w1538 w1634 w1712 w1766] -> w166
      tunnel: [w213 w247 w283 w388 w479 w547 w642 w786 w863 w940 w981 w1024 w1064 w1087 w1127 w1153 w1200 w1245 w1325 w1387 w1424 w1482 w1539 w1635 w1713 w1767] -> w165
      tunnel: w164 -> [_ _ _ w383 w476 _ w635 w781 _ _ _ _ _ _ _ _ _ _ _ _ _ _ _ _ _ _]
      tunnel: w163 -> [_ _ _ w381 w475 _ _ _ _ _ _ _ _ _ _ _ _ _ _ _ _ _ _ _ _ _]
      tunnel: [w212 w243 w276 w313 w452 w537 w632 w712 w849 w935 w975 w1018 w1050 w1085 w1120 w1152 w1181 w1234 w1291 w1378 w1410 w1472 w1530 w1586 w1668 w1756] -> w77
      tunnel: w162 -> [w212 w243 w276 w378 w452 w537 w632 w777 w849 w935 w975 w1018 w1050 w1085 w1120 w1152 w1181 w1234 w1291 w1378 w1410 w1472 w1530 w1586 w1668 w1756]
      tunnel: w129 -> [_ _ _ w375 w449 w535 w630 w774 w846 _ _ _ _ _ _ _ w1179 w1232 w1304 _ w1407 w1469 w1527 w1583 w1664 _]
      tunnel: w160 -> [_ _ _ w372 w448 w533 w629 w771 w845 _ _ _ _ _ _ _ w1177 w1230 w1303 _ w1406 w1468 w1526 w1582 w1665 _]
      tunnel: w112 -> [_ _ _ w367 _ _ _ w766 _ _ _ _ _ _ _ _ _ _ _ _ _ _ _ _ _ _]
      tunnel: [w211 w242 w275 w321 w451 w536 w631 w720 w848 w934 w974 w1017 w1049 w1084 w1119 w1151 w1180 w1233 w1306 w1377 w1409 w1471 w1529 w1585 w1667 w1762] -> w113
      tunnel: w158 -> [w211 w242 w275 w371 w451 w536 w631 w770 w848 w934 w974 w1017 w1049 w1084 w1119 w1151 w1180 w1233 w1306 w1377 w1409 w1471 w1529 w1585 w1667 w1762]
      tunnel: [w210 w241 w274 w312 w447 w532 w628 w711 w844 w933 w973 w1016 w1048 w1083 w1118 w1150 w1176 w1229 w1290 w1376 w1405 w1467 w1525 w1581 w1663 w1751] -> w76
      tunnel: w134 -> [w210 w241 w274 w365 w447 w532 w628 w764 w844 w933 w973 w1016 w1048 w1083 w1118 w1150 w1176 w1229 w1290 w1376 w1405 w1467 w1525 w1581 w1663 w1751]
      tunnel: [w209 w240 w273 w358 w446 w531 w618 w757 w843 w932 w972 w1015 w1047 w1082 w1117 w1149 w1175 w1228 w1302 w1375 w1404 w1466 w1524 w1580 w1662 w1750] -> w107
      tunnel: w120 -> [w209 w240 w273 w358 w446 w531 w618 w757 w843 w932 w972 w1015 w1047 w1082 w1117 w1149 w1175 w1228 w1302 w1375 w1404 w1466 w1524 w1580 w1662 w1749]
      tunnel: [w208 w239 w272 w357 w445 w530 w617 w756 w842 w931 w971 w1014 w1046 w1081 w1116 w1148 w1174 w1227 w1301 w1374 w1403 w1465 w1523 w1579 w1661 w1735] -> w115
      tunnel: w114 -> [w208 w239 w272 w357 w445 w530 w617 w756 w842 w931 w971 w1014 w1046 w1081 w1116 w1148 w1174 w1227 w1301 w1374 w1403 w1465 w1523 w1579 w1661 w1735]
      tunnel: w112 -> [_ _ _ _ _ _ _ _ _ _ _ _ _ _ _ _ _ _ _ _ _ _ _ _ _ _]
      tunnel: [w207 w238 w271 w356 w444 w529 w616 w755 w841 w930 w970 w1013 w1045 w1080 w1115 w1147 w1173 w1226 w1300 w1373 w1402 w1464 w1522 w1578 w1660 w1734] -> w108
      tunnel: w110 -> [w207 w238 w271 w356 w444 w529 w616 w755 w841 w930 w970 w1013 w1045 w1080 w1115 w1147 w1173 w1226 w1300 w1373 w1402 w1464 w1522 w1578 w1660 w1734]
      tunnel: [w205 w236 w269 w306 w441 w527 w614 w705 w839 w928 w969 w1012 w1043 w1078 w1113 w1145 w1171 w1225 w1299 w1372 w1401 w1463 w1520 w1577 w1659 w1733] -> w70
      tunnel: w98 -> [w205 w236 w269 w352 w441 w527 w614 w751 w839 w928 w969 w1012 w1043 w1078 w1113 w1145 w1171 w1225 w1299 w1372 w1401 w1463 w1520 w1577 w1659 w1733]
      tunnel: [w206 w237 w270 w307 w442 w528 w615 w706 w840 w929 w968 w1011 w1044 w1079 w1114 w1146 w1172 w1224 w1298 w1371 w1400 w1462 w1521 w1576 w1658 w1732] -> w71
      tunnel: w97 -> [w206 w237 w270 w351 w442 w528 w615 w750 w840 w929 w968 w1011 w1044 w1079 w1114 w1146 w1172 w1224 w1298 w1371 w1400 w1462 w1521 w1576 w1658 w1732]
      tunnel: [w198 w229 w262 w311 w438 w525 w612 w710 w837 w921 w966 w1009 w1041 w1076 w1111 w1143 w1164 w1217 w1289 w1370 w1393 w1455 w1513 w1569 w1653 w1725] -> w75
      tunnel: w86 -> [w198 w229 w262 w341 w438 w525 w612 w740 w837 w921 w966 w1009 w1041 w1076 w1111 w1143 w1164 w1217 w1289 w1370 w1393 w1455 w1513 w1569 w1653 w1725]
      tunnel: [w197 w228 w261 w310 w439 w526 w613 w709 w838 w920 w967 w1010 w1042 w1077 w1112 w1144 w1163 w1216 w1288 w1369 w1392 w1454 w1512 w1568 w1652 w1724] -> w74
      tunnel: w85 -> [w197 w228 w261 w340 w439 w526 w613 w739 w838 w920 w967 w1010 w1042 w1077 w1112 w1144 w1163 w1216 w1288 w1369 w1392 w1454 w1512 w1568 w1652 w1724]
      tunnel: [w200 w231 w264 w316 w437 w523 w610 w715 w835 w926 w964 w1007 w1039 w1074 w1109 w1141 w1166 w1219 w1293 w1364 w1395 w1457 w1515 w1571 w1651 w1729] -> w68
      tunnel: w84 -> [w200 w231 w264 w337 w437 w523 w610 w736 w835 w926 w964 w1007 w1039 w1074 w1109 w1141 w1166 w1219 w1293 w1364 w1395 w1457 w1515 w1571 w1651 w1729]
      tunnel: [w199 w230 w263 w314 w440 w524 w611 w713 w836 w927 w965 w1008 w1040 w1075 w1110 w1142 w1165 w1218 w1292 w1363 w1394 w1456 w1514 w1570 w1650 w1728] -> w78
      tunnel: w83 -> [w199 w230 w263 w336 w440 w524 w611 w735 w836 w927 w965 w1008 w1040 w1075 w1110 w1142 w1165 w1218 w1292 w1363 w1394 w1456 w1514 w1570 w1650 w1728]
      tunnel: [w202 w233 w266 w305 w436 w521 w608 w704 w833 w924 w962 w1005 w1037 w1072 w1107 w1139 w1168 w1221 w1295 w1366 w1397 w1459 w1517 w1573 w1655 w1731] -> w69
      tunnel: w82 -> [w202 w233 w266 w333 w436 w521 w608 w732 w833 w924 w962 w1005 w1037 w1072 w1107 w1139 w1168 w1221 w1295 w1366 w1397 w1459 w1517 w1573 w1655 w1731]
      tunnel: [w201 w232 w265 w304 w435 w522 w609 w703 w834 w925 w963 w1006 w1038 w1073 w1108 w1140 w1167 w1220 w1294 w1365 w1396 w1458 w1516 w1572 w1654 w1730] -> w67
      tunnel: w81 -> [w201 w232 w265 w332 w435 w522 w609 w731 w834 w925 w963 w1006 w1038 w1073 w1108 w1140 w1167 w1220 w1294 w1365 w1396 w1458 w1516 w1572 w1654 w1730]
      tunnel: [w204 w235 w268 w309 w434 w519 w606 w708 w831 w922 w960 w1003 w1035 w1070 w1105 w1137 w1170 w1223 w1297 w1368 w1399 w1461 w1519 w1575 w1657 w1727] -> w73
      tunnel: w80 -> [w204 w235 w268 w329 w434 w519 w606 w728 w831 w922 w960 w1003 w1035 w1070 w1105 w1137 w1170 w1223 w1297 w1368 w1399 w1461 w1519 w1575 w1657 w1727]
      tunnel: [w203 w234 w267 w308 w433 w520 w607 w707 w832 w923 w961 w1004 w1036 w1071 w1106 w1138 w1169 w1222 w1296 w1367 w1398 w1460 w1518 w1574 w1656 w1726] -> w72
      tunnel: w79 -> [w203 w234 w267 w328 w433 w520 w607 w727 w832 w923 w961 w1004 w1036 w1071 w1106 w1138 w1169 w1222 w1296 w1367 w1398 w1460 w1518 w1574 w1656 w1726]
      frame "wait" {
        n32 = Index Array(array=w227, index=0 ("Index")) -> (element=w225:string)
        n33 = Decimal String To Number(string=w225, default (0L)=u32 0) -> (number=w224:u32)  [unwired: 1 in, 1 out]
        n34 = Wait (ms)(milliseconds to wait=w224) -> ()  [unwired: 1 out]
      }
      frame "wait-min" {
        n35 = Index Array(array=w260, index=0 ("Index")) -> (element=w258:string)
        n36 = Decimal String To Number(string=w258, default (0L)=u32 0) -> (number=w246:u32)  [unwired: 1 in, 1 out]
        n37 = Multiply(x=w246, y=u32 60000) -> (x*y=w245:u32)
        n38 = Wait (ms)(milliseconds to wait=w245) -> ()  [unwired: 1 out]
      }
      frame "standby" {
        n39 = Index Array(array=w292, index=0 ("Index")) -> (element=w282:string)
        n40 = case shown="\"off\", Default" w282 {
          tunnel: [":PAGE:SCON:STAN 0" ":PAGE:SCON:STAN 1"] -> w277
          frame "off", Default {
          }
          frame "on" {
          }
        }
        n41 = VISA Write(VISA resource name=w281, write buffer=w277, error in (no error)=w280) -> (VISA resource name out=w279:refnum<visa-resource-name>, error out=w278:errorcluster)  [unwired: 1 out]
      }
      frame "transfer" {
        # "Adjusts graph colors."
        # "Adjusts graph colors."
        # "Is off"
        # "Is on"
        # "Ion will be the middle element of the array. The calculation of the index is done only once, since Is, Id, and Ig have the same dimensions."
        # "Ig off"
        # "Ig on"
        # "Is min"
        # "Is max"
        # "Ig min"
        # "Ig max"
        # "abs(Ig)"
        # "abs(Is)"
        # "Id min"
        # "Id max"
        # "Y1: Is\nY2: Id\nY3: Ig"
        # "abs(Id)"
        # "Adjusts graph colors."
        # "Adjusts graph colors."
        # "Id off"
        # "Id on"
        # "Adjusts graph colors."
        # "Time array"
        n42 = Delete From Array(array=w420, index=0 ("Index")) -> (deleted portion=w418:string, array with subset deleted=w417:string[])  [unwired: 1 in]
        n43 = Bundle By Name(cluster=w381, "Emergency Stop"=w429) -> (w382:T3)
        n44 = Number To Decimal String(number=w375) -> (decimal integer string=w374:string)  [unwired: 1 in]
        n45 = case shown="\"d\", Default" w418 {
          tunnel: [w431 w432] -> w416
          frame "s" {
            w431 = u16 0 items=["Single", "Double"] ("sweep mode")
          }
          frame "d", Default {
            w432 = u16 1 items=["Single", "Double"] ("sweep mode")
          }
        }
        n46 = Fract/Exp String To Number(string=w417) -> (number=w402:dbl[])  [unwired: 3 in, 1 out]
        n47 = Concatenate Strings(w427, "-transfer-" ("Prefix"), w374, w372, ".txt" ("Suffix (transfer)")) -> (w428:string)
        n48 = VISA Write(VISA resource name=w398, write buffer=":PAGE:CHAN:MODE SWE;" ("write buffer (\"\")"), error in (no error)=w397) -> (VISA resource name out=w395:refnum<visa-resource-name>, error out=w396:errorcluster)  [unwired: 1 out]
        n49 = String To Path(string=w428) -> (path=w426:path)
        n50 = Index Array(array=w402, index #1=0 ("Index")) -> (element #1=w415:dbl, element #2=w414:dbl, element #3=w413:dbl)  [unwired: 2 in]
        n51 = Delete From Array(array=w402, length=3 ("Length"), index=0 ("Index")) -> (array with subset deleted=w400:dbl[])  [unwired: 1 out]
        n52 = Build Array (concatenate)(w371, w367) -> (w321:i32[])
        n53 = Bundle By Name(cluster=w407, "Gate Start"=w415, "Gate Stop"=w414, "Gate Step (linear only)"=w413, "Gate Compliance"=w424, "Range mode"=w391, "Range"=w390) -> (w392:T6)
        n54 = control-ref of="Imax vs time"() -> (w350:refnum<vi>)
        n55 = control-ref of="Imin vs time"() -> (w349:refnum<vi>)
        n56 = control-ref of="Ion vs time"() -> (w318:refnum<vi>)
        n57 = control-ref of="Ioff vs time"() -> (w317:refnum<vi>)
        n58 = control-ref of="I vs Vg"() -> (w376:refnum<vi>)
        n59 = Index Array(array=w400, index #1=0 ("Index")) -> (element #1=w410:dbl, element #2=w409:dbl, element #3=w408:dbl)  [unwired: 2 in]
        n60 = call <vilib>:"compatOverwrite.vi"("overwrite (F)"=TRUE) -> ("overwrite?"=w380:T8)
        n61 = Bundle By Name(cluster=w406, "Drain Start"=w410, "Drain Stop"=w409, "Drain Step"=w408, "Drain Compliance"=w425, "Range mode"=w389, "Range"=w388) -> (w393:T7)
        n62 = call "4155C Transfer.vi"("VISA resource name in"=w395, "Gate"=w392, "Drain"=w393, "Timings"=w423, "error in (no error)"=w396, "SMU4"=w383, "sweep mode"=w416, "Panel Controls"=w382) -> ("VG"=w379:dbl[], "Outparams"=w387:T9, "VISA Resource Name out"=w422:refnum<visa-resource-name>, "IS"=w346:dbl[], "ID"=w348:dbl[], "IG"=w345:dbl[], "error out"=w368:errorcluster, "SMU4"=w384:dbl[])  [unwired: 12 in]
        n63 = Unbundle By Name(w387) -> ("V2 Step"=w386:dbl, "V2 Start"=w385:dbl, "Number of points"=w315:i32)
        n64 = Absolute Value(x=w346) -> (abs(x)=w331:dbl[])
        n65 = Absolute Value(x=w348) -> (abs(x)=w347:dbl[])
        n66 = Absolute Value(x=w345) -> (abs(x)=w334:dbl[])
        n67 = Array Size(array=w347) -> (size(s)=w355:i32)
        n68 = Divide(x=w355, y=2) -> (x/y=w298:dbl)
        n69 = Subtract(x=w298, y=1) -> (x-y=w297:dbl)
        n70 = Array Max & Min(array=w331) -> (max value=w338:dbl, min value=w339:dbl)  [unwired: 2 out]
        n71 = Array Max & Min(array=w347) -> (max value=w377:dbl, min value=w344:dbl)  [unwired: 2 out]
        n72 = Array Max & Min(array=w334) -> (max value=w343:dbl, min value=w342:dbl)  [unwired: 2 out]
        n73 = call "4155C Split array.vi"("Number of VAR2 steps"=w315, "Y2 data in"=w348, "X data in"=w379, "Y1 data in"=w346, "Y3 data in"=w345, "error in (no error)"=w368) -> ("Array of clusters"=w370:cluster{"Y data in":dbl[], "X data in":dbl[]}[], "error out"=w303:errorcluster)  [unwired: 1 in]
        n74 = Index Array(array=w331, index=w297) -> (element=w322:dbl)
        n75 = Index Array(array=w331, index=0) -> (element=w323:dbl)
        n76 = Index Array(array=w347, index=w297) -> (element=w324:dbl)
        n77 = Index Array(array=w347, index=0) -> (element=w325:dbl)
        n78 = Index Array(array=w334, index=w297) -> (element=w327:dbl)
        n79 = Index Array(array=w334, index=0) -> (element=w326:dbl)
        n80 = local write "Ig max"(w343) -> ()
        n81 = local write "Ig min"(w342) -> ()
        n82 = local write "Is max"(w338) -> ()
        n83 = local write "Is min"(w339) -> ()
        n84 = local write "Id max"(w377) -> ()
        n85 = local write "Id min"(w344) -> ()
        n86 = local write "I vs Vg"(w370) -> ()
        n87 = Build Array (concatenate)(w337, w338) -> (w316:dbl[])
        n88 = Build Array (concatenate)(w336, w339) -> (w314:dbl[])
        n89 = local write "Is off"(w323) -> ()
        n90 = local write "Is on"(w322) -> ()
        n91 = Build Array (concatenate)(w378, w377) -> (w313:dbl[])
        n92 = Build Array (concatenate)(w365, w344) -> (w312:dbl[])
        n93 = Build Array (concatenate)(w341, w343) -> (w311:dbl[])
        n94 = Build Array (concatenate)(w340, w342) -> (w310:dbl[])
        n95 = Build Array (concatenate)(w329, w322) -> (w309:dbl[])
        n96 = Build Array (concatenate)(w328, w323) -> (w308:dbl[])
        n97 = Build Array (concatenate)(w351, w324) -> (w307:dbl[])
        n98 = Build Array (concatenate)(w352, w325) -> (w306:dbl[])
        n99 = Build Array (concatenate)(w333, w327) -> (w305:dbl[])
        n100 = Build Array (concatenate)(w332, w326) -> (w304:dbl[])
        n101 = local write "Ig off"(w326) -> ()
        n102 = local write "Ig on"(w327) -> ()
        n103 = local write "Id off"(w325) -> ()
        n104 = local write "Id on"(w324) -> ()
        n105 = call "4155C Split array.vi"("Number of VAR2 steps"=w315, "Y2 data in"=w307, "X data in"=w321, "Y1 data in"=w309, "Y3 data in"=w305, "error in (no error)"=w303) -> ("Array of clusters"=w319:cluster{"Y data in":dbl[], "X data in":dbl[]}[], "error out"=w302:errorcluster)  [unwired: 1 in]
        n106 = call "4155C Split array.vi"("Number of VAR2 steps"=w315, "Y2 data in"=w306, "X data in"=w321, "Y1 data in"=w308, "Y3 data in"=w304, "error in (no error)"=w302) -> ("Array of clusters"=w320:cluster{"Y data in":dbl[], "X data in":dbl[]}[], "error out"=w301:errorcluster)  [unwired: 1 in]
        n107 = call "4155C Split array.vi"("Number of VAR2 steps"=w315, "Y2 data in"=w313, "X data in"=w321, "Y1 data in"=w316, "Y3 data in"=w311, "error in (no error)"=w301) -> ("Array of clusters"=w369:cluster{"Y data in":dbl[], "X data in":dbl[]}[], "error out"=w300:errorcluster)  [unwired: 1 in]
        n108 = call "4155C Split array.vi"("Number of VAR2 steps"=w315, "Y2 data in"=w312, "X data in"=w321, "Y1 data in"=w314, "Y3 data in"=w310, "error in (no error)"=w300) -> ("Array of clusters"=w366:cluster{"Y data in":dbl[], "X data in":dbl[]}[], "error out"=w299:errorcluster)  [unwired: 1 in]
        n109 = Open/Create/Replace File(file path (use dialog)=w426, error in=w299, operation (0:open)=w380) -> (refnum out=w363:refnum<file>, error out=w361:errorcluster)  [unwired: 3 in, 1 out]
        n110 = call "4155C Make Big 2d array.vi"("1D Var1"=w379, "1d IS"=w346, "1d ID"=w348, "1d IG"=w345, "1d SMU4"=w384, "SMU4"=w383, "VAR2 START"=w385, "Number of VAR2 steps"=w315, "VAR2 STEP"=w386, "VAR1 Name"="Vg", "Decimal places in header"=i8 1, "VAR2 Name"="Vd") -> ("Header array"=w364:string[], "Data array"=w362:dbl[][])  [unwired: 14 in]
        n111 = local write "Imax vs time"(w369) -> ()
        n112 = local write "Imin vs time"(w366) -> ()
        n113 = local write "Ion vs time"(w319) -> ()
        n114 = local write "Ioff vs time"(w320) -> ()
        n115 = call "4155C Config Chart Colours.vi"("Numeric"=w315, "XY Graph 2"=w350) -> ()  [unwired: 6 in]
        n116 = call "4155C Config Chart Colours.vi"("Numeric"=w315, "XY Graph 2"=w349) -> ()  [unwired: 6 in]
        n117 = call "4155C Config Chart Colours.vi"("Numeric"=w315, "XY Graph 2"=w318) -> ()  [unwired: 6 in]
        n118 = call "4155C Config Chart Colours.vi"("Numeric"=w315, "XY Graph 2"=w317) -> ()  [unwired: 6 in]
        n119 = call "4155C Config Chart Colours.vi"("Numeric"=w315, "XY Graph 2"=w376) -> ()  [unwired: 6 in]
        n120 = call "4155C Write array to file.vi"("Byte Stream File Refnum"=w363, "Header"=w364, "Data Array"=w362, "error in (no error)"=w361) -> ("dup refnum"=w360:refnum<file>, "error out"=w359:errorcluster)  [unwired: 1 in]
        n121 = Close File(refnum=w360, error in=w359) -> (error out=w421:errorcluster)  [unwired: 1 out]
      }
      frame "pulsedstressV" {
        w458 = 0
        n122 = Number To Decimal String(number=w449) -> (decimal integer string=w505:string)  [unwired: 1 in]
        n123 = Delete From Array(array=w443, index=0 ("Index")) -> (deleted portion=w496:string, array with subset deleted=w495:string[])  [unwired: 1 in]
        n124 = Bundle By Name(cluster=w475, "Emergency Stop"=w508) -> (w477:T3)
        n125 = VISA Write(VISA resource name=w489, write buffer=":PAGE:CHAN:MODE SWE;" ("write buffer (\"\")"), error in (no error)=w488) -> (VISA resource name out=w486:refnum<visa-resource-name>, error out=w487:errorcluster)  [unwired: 1 out]
        n126 = Concatenate Strings(w504, "-pulsedstressV-" ("Substring"), w505, w448, ".txt" ("Substring")) -> (w507:string)
        n127 = case shown="\"d\", Default" w496 {
          tunnel: [w517 w518] -> w494
          frame "s" {
            w517 = u16 0 items=["Single", "Double"] ("sweep mode")
          }
          frame "d", Default {
            w518 = u16 1 items=["Single", "Double"] ("sweep mode")
          }
        }
        n128 = Fract/Exp String To Number(string=w495) -> (number=w490:dbl[])  [unwired: 3 in, 1 out]
        n129 = String To Path(string=w507) -> (path=w503:path)
        n130 = Index Array(array=w490, index #1=0 ("Index")) -> (element #1=w467:dbl, element #2=w466:dbl, element #3=w463:dbl, element #4=w462:dbl, element #5=w461:dbl, element #6=w465:dbl)  [unwired: 5 in]
        n131 = Bundle By Name(cluster=w464, "Pulse period"=w462, "Base voltage"=w463, "Pulse width"=w461) -> (w460:T5)
        n132 = Unbundle By Name(w460) -> ("Pulse period"=w468:dbl)
        n133 = Bundle By Name(cluster=w492, "Gate Start"=w466, "Gate Stop"=w467, "Gate Step (linear only)"=0, "Gate Compliance"=w501, "Range mode"=w482, "Range"=w481) -> (w483:T6)
        n134 = call <vilib>:"compatOverwrite.vi"("overwrite (F)"=TRUE) -> ("overwrite?"=w453:T8)
        n135 = Bundle By Name(cluster=w491, "Drain Start"=w465, "Drain Stop"=w458, "Drain Step"=w458, "Drain Compliance"=w502, "Range mode"=w480, "Range"=w479) -> (w484:T7)
        n136 = call "4155C PulsedStressV.vi"("VISA resource name in"=w486, "sweep mode"=w494, "Panel Controls"=w477, "Gate"=w483, "Drain"=w484, "Timings"=w460, "error in (no error)"=w487, "SMU4"=w476) -> ("VISA Resource Name out"=w499:refnum<visa-resource-name>, "ID"=w456:dbl[], "IG"=w454:dbl[], "Outparams"=w478:T9, "error out"=w500:errorcluster)  [unwired: 3 in]
        n137 = Unbundle By Name(w478) -> ("Number of points"=w455:i32)  [unwired: 2 out]
        n138 = for {
          N: w455 -> [_]
          tunnel: [w514] -> w457 mode=indexing
          tunnel: w468 -> [w516]
          i -> [w515]
          n139 = Multiply(x=w516, y=w515) -> (x*y=w514:dbl)
        }
        n140 = Insert Into Array(array=dbl[][] [] ("Input Array"), new element=w457) -> (w469:dbl[][])  [unwired: 2 in]
        n141 = Insert Into Array(array=w469, new element=w456) -> (w474:dbl[][])  [unwired: 2 in]
        n142 = Insert Into Array(array=w474, new element=w454) -> (w473:dbl[][])  [unwired: 2 in]
        n143 = Transpose 2D Array(2D array=w473) -> (transposed array=w472:dbl[][])
        n144 = Open/Create/Replace File(file path (use dialog)=w503, error in=w500, operation (0:open)=w453) -> (refnum out=w511:refnum<file>, error out=w512:errorcluster)  [unwired: 3 in, 1 out]
        n145 = call "4155C Write array to file.vi"("Byte Stream File Refnum"=w511, "Header"=string[] ["Time /s", "Id /A", "Ig /A"], "Data Array"=w472, "error in (no error)"=w512) -> ("dup refnum"=w509:refnum<file>, "error out"=w510:errorcluster)  [unwired: 1 in]
        n146 = Close File(refnum=w509, error in=w510) -> (error out=w498:errorcluster)  [unwired: 1 out]
      }
      frame "transfer-fpp" {
        n147 = Number To Decimal String(number=w535) -> (decimal integer string=w589:string)  [unwired: 1 in]
        n148 = Bundle By Name(cluster=w565, "Emergency Stop"=w593) -> (w601:T2)
        n149 = Delete From Array(array=w580, index=0 ("Index")) -> (deleted portion=w578:string, array with subset deleted=w577:string[])  [unwired: 1 in]
        n150 = Concatenate Strings(w588, "-transferfpp-" ("Substring"), w589, w533, ".txt" ("Substring")) -> (w591:string)
        n151 = VISA Write(VISA resource name=w557, write buffer=":PAGE:CHAN:MODE SWE;" ("write buffer (\"\")"), error in (no error)=w556) -> (VISA resource name out=w554:refnum<visa-resource-name>, error out=w555:errorcluster)  [unwired: 1 out]
        n152 = case shown="\"d\", Default" w578 {
          tunnel: [w602 w603] -> w576
          frame "s" {
            w602 = u16 0 items=["Single", "Double"] ("sweep mode")
          }
          frame "d", Default {
            w603 = u16 1 items=["Single", "Double"] ("sweep mode")
          }
        }
        n153 = Fract/Exp String To Number(string=w577) -> (number=w561:dbl[])  [unwired: 3 in, 1 out]
        n154 = String To Path(string=w591) -> (path=w587:path)
        n155 = Index Array(array=w561, index #1=0 ("Index")) -> (element #1=w575:dbl, element #2=w574:dbl, element #3=w573:dbl)  [unwired: 2 in]
        n156 = Delete From Array(array=w561, length=3 ("Length"), index=0 ("Index")) -> (array with subset deleted=w559:dbl[])  [unwired: 1 out]
        n157 = Bundle By Name(cluster=w567, "Gate Start"=w575, "Gate Stop"=w574, "Gate Step (linear only)"=w573, "Gate Compliance"=w585, "Range mode"=w550, "Range"=w549) -> (w551:T6)
        n158 = Index Array(array=w559, index #1=0 ("Index")) -> (element #1=w570:dbl, element #2=w569:dbl, element #3=w568:dbl)  [unwired: 2 in]
        n159 = call <vilib>:"compatOverwrite.vi"("overwrite (F)"=TRUE) -> ("overwrite?"=w538:T8)
        n160 = Bundle By Name(cluster=w566, "Drain Start"=w570, "Drain Stop"=w569, "Drain Step"=w568, "Drain Compliance"=w586, "Range mode"=w548, "Range"=w547) -> (w552:T7)
        n161 = call "4155C Transfer-FPP.vi"("VISA resource name in"=w554, "Gate"=w551, "Drain"=w552, "Timings"=w584, "error in (no error)"=w555, "sweep mode"=w576, "Panel Controls"=w601) -> ("VG"=w592:dbl[], "Outparams"=w546:T9, "VISA Resource Name out"=w582:refnum<visa-resource-name>, "Vprobe2"=w542:dbl[], "ID"=w541:dbl[], "IG"=w540:dbl[], "Vprobe1"=w539:dbl[], "error out"=w583:errorcluster)  [unwired: 13 in]
        n162 = Unbundle By Name(w546) -> ("V2 Step"=w545:dbl, "V2 Start"=w544:dbl, "Number of points"=w543:i32)
        n163 = Open/Create/Replace File(file path (use dialog)=w587, error in=w583, operation (0:open)=w538) -> (refnum out=w598:refnum<file>, error out=w599:errorcluster)  [unwired: 3 in, 1 out]
        n164 = call "4155C Make Big 2d array FPP.vi"("1D Var1"=w592, "1d ID"=w541, "1d Vp2"=w542, "1d IG"=w540, "1d Vp1"=w539, "VAR2 START"=w544, "Number of VAR2 steps"=w543, "VAR2 STEP"=w545, "VAR1 Name"="Vg", "Decimal places in header"=i8 1, "VAR2 Name"="Vd") -> ("Header array"=w594:string[], "Data array"=w595:dbl[][])  [unwired: 15 in]
        n165 = call "4155C Write array to file.vi"("Byte Stream File Refnum"=w598, "Header"=w594, "Data Array"=w595, "error in (no error)"=w599) -> ("dup refnum"=w596:refnum<file>, "error out"=w597:errorcluster)  [unwired: 1 in]
        n166 = Close File(refnum=w596, error in=w597) -> (error out=w581:errorcluster)  [unwired: 1 out]
      }
      frame "output" {
        n167 = Number To Decimal String(number=w630) -> (decimal integer string=w678:string)  [unwired: 1 in]
        n168 = Bundle By Name(cluster=w655, "Emergency Stop"=w680) -> (w690:T2)
        n169 = Delete From Array(array=w670, index=0 ("Index")) -> (deleted portion=w668:string, array with subset deleted=w667:string[])  [unwired: 1 in]
        n170 = Concatenate Strings(w677, "-output-" ("Substring"), w678, w629, ".txt" ("Suffix (output)")) -> (w679:string)
        n171 = VISA Write(VISA resource name=w646, write buffer=":PAGE:CHAN:MODE SWE;" ("write buffer (\"\")"), error in (no error)=w643) -> (VISA resource name out=w645:refnum<visa-resource-name>, error out=w644:errorcluster)  [unwired: 1 out]
        n172 = case shown="\"d\", Default" w668 {
          tunnel: [w691 w692] -> w666
          frame "s" {
            w691 = u16 0 items=["Single", "Double"] ("sweep mode")
          }
          frame "d", Default {
            w692 = u16 1 items=["Single", "Double"] ("sweep mode")
          }
        }
        n173 = Fract/Exp String To Number(string=w667) -> (number=w649:dbl[])  [unwired: 3 in, 1 out]
        n174 = String To Path(string=w679) -> (path=w676:path)
        n175 = Index Array(array=w649, index #1=0 ("Index")) -> (element #1=w665:dbl, element #2=w664:dbl, element #3=w663:dbl)  [unwired: 2 in]
        n176 = Delete From Array(array=w649, length=3 ("Length"), index=0 ("Index")) -> (array with subset deleted=w648:dbl[])  [unwired: 1 out]
        n177 = control-ref of="I vs Vd"() -> (w620:refnum<vi>)
        n178 = Bundle By Name(cluster=w657, "Gate Start"=w665, "Gate Stop"=w664, "Gate Step (linear only)"=w663, "Gate Compliance"=w674, "Range mode"=w641, "Range"=w640) -> (w689:T6)
        n179 = Index Array(array=w648, index #1=0 ("Index")) -> (element #1=w660:dbl, element #2=w659:dbl, element #3=w658:dbl)  [unwired: 2 in]
        n180 = call <vilib>:"compatOverwrite.vi"("overwrite (F)"=TRUE) -> ("overwrite?"=w633:T8)
        n181 = Bundle By Name(cluster=w656, "Drain Start"=w660, "Drain Stop"=w659, "Drain Step"=w658, "Drain Compliance"=w675, "Range mode"=w639, "Range"=w642) -> (w688:T7)
        n182 = call "4155C Output.vi"("VISA resource name in"=w645, "Gate"=w689, "Drain"=w688, "Timings"=w673, "error in (no error)"=w644, "SMU4"=w635, "sweep mode"=w666, "Panel controls"=w690) -> ("VD"=w627:dbl[], "Outparams"=w637:T9, "VISA Resource Name out"=w672:refnum<visa-resource-name>, "IS"=w626:dbl[], "ID"=w625:dbl[], "IG"=w624:dbl[], "error out"=w622:errorcluster, "SMU4"=w634:dbl[])  [unwired: 12 in]
        n183 = Unbundle By Name(w637) -> ("V2 Step"=w638:dbl, "V2 Start"=w636:dbl, "Number of points"=w619:i32)
        n184 = call "4155C Split array.vi"("Number of VAR2 steps"=w619, "Y2 data in"=w625, "X data in"=w627, "Y1 data in"=w626, "Y3 data in"=w624, "error in (no error)"=w622) -> ("Array of clusters"=w623:cluster{"Y data in":dbl[], "X data in":dbl[]}[], "error out"=w621:errorcluster)  [unwired: 1 in]
        n185 = local write "I vs Vd"(w623) -> ()
        n186 = call "4155C Config Chart Colours.vi"("Numeric"=w619, "XY Graph 2"=w620) -> ()  [unwired: 6 in]
        n187 = Open/Create/Replace File(file path (use dialog)=w676, error in=w621, operation (0:open)=w633) -> (refnum out=w685:refnum<file>, error out=w686:errorcluster)  [unwired: 3 in, 1 out]
        n188 = call "4155C Make Big 2d array.vi"("1D Var1"=w627, "1d IS"=w626, "1d ID"=w625, "1d IG"=w624, "1d SMU4"=w634, "SMU4"=w635, "VAR2 START"=w636, "Number of VAR2 steps"=w619, "VAR2 STEP"=w638, "VAR1 Name"="Vd", "Decimal places in header"=i8 1, "VAR2 Name"="Vg") -> ("Header array"=w681:string[], "Data array"=w682:dbl[][])  [unwired: 14 in]
        n189 = call "4155C Write array to file.vi"("Byte Stream File Refnum"=w685, "Header"=w681, "Data Array"=w682, "error in (no error)"=w686) -> ("dup refnum"=w683:refnum<file>, "error out"=w684:errorcluster)  [unwired: 1 in]
        n190 = Close File(refnum=w683, error in=w684) -> (error out=w671:errorcluster)  [unwired: 1 out]
      }
      frame "output2" {
        # "Adjusts graph colors."
        # "Adjusts graph colors."
        # "Is off"
        # "Is on"
        # "Ion will be the middle element of the array. The calculation of the index is done only once, since Is, Id, and Ig have the same dimensions."
        # "Ig off"
        # "Ig on"
        # "Is min"
        # "Is max"
        # "Ig min"
        # "Ig max"
        # "abs(Ig)"
        # "abs(Is)"
        # "Id min"
        # "Id max"
        # "Y1: Is\nY2: Id\nY3: Ig"
        # "abs(Id)"
        # "Adjusts graph colors."
        # "Adjusts graph colors."
        # "Id off"
        # "Id on"
        # "Adjusts graph colors."
        # "Time array"
        n191 = Delete From Array(array=w818, index=0 ("Index")) -> (deleted portion=w816:string, array with subset deleted=w815:string[])  [unwired: 1 in]
        n192 = Bundle By Name(cluster=w694, "Emergency Stop"=w827) -> (w780:T2)
        n193 = Number To Decimal String(number=w774) -> (decimal integer string=w773:string)  [unwired: 1 in]
        n194 = case shown="\"d\", Default" w816 {
          tunnel: [w829 w830] -> w814
          frame "s" {
            w829 = u16 0 items=["Single", "Double"] ("sweep mode")
          }
          frame "d", Default {
            w830 = u16 1 items=["Single", "Double"] ("sweep mode")
          }
        }
        n195 = Fract/Exp String To Number(string=w815) -> (number=w800:dbl[])  [unwired: 3 in, 1 out]
        n196 = Concatenate Strings(w825, "-output-" ("Substring"), w773, w771, ".txt" ("Suffix (transfer)")) -> (w826:string)
        n197 = VISA Write(VISA resource name=w796, write buffer=":PAGE:CHAN:MODE SWE;" ("write buffer (\"\")"), error in (no error)=w795) -> (VISA resource name out=w793:refnum<visa-resource-name>, error out=w794:errorcluster)  [unwired: 1 out]
        n198 = String To Path(string=w826) -> (path=w824:path)
        n199 = Index Array(array=w800, index #1=0 ("Index")) -> (element #1=w813:dbl, element #2=w812:dbl, element #3=w811:dbl)  [unwired: 2 in]
        n200 = Delete From Array(array=w800, length=3 ("Length"), index=0 ("Index")) -> (array with subset deleted=w798:dbl[])  [unwired: 1 out]
        n201 = Build Array (concatenate)(w770, w766) -> (w720:i32[])
        n202 = Bundle By Name(cluster=w805, "Gate Start"=w813, "Gate Stop"=w812, "Gate Step (linear only)"=w811, "Gate Compliance"=w822, "Range mode"=w789, "Range"=w788) -> (w790:T6)
        n203 = control-ref of="Imax vs time"() -> (w749:refnum<vi>)
        n204 = control-ref of="Imin vs time"() -> (w748:refnum<vi>)
        n205 = control-ref of="Ion vs time"() -> (w717:refnum<vi>)
        n206 = control-ref of="Ioff vs time"() -> (w716:refnum<vi>)
        n207 = control-ref of="I vs Vg"() -> (w775:refnum<vi>)
        n208 = Index Array(array=w798, index #1=0 ("Index")) -> (element #1=w808:dbl, element #2=w807:dbl, element #3=w806:dbl)  [unwired: 2 in]
        n209 = call <vilib>:"compatOverwrite.vi"("overwrite (F)"=TRUE) -> ("overwrite?"=w779:T8)
        n210 = Bundle By Name(cluster=w804, "Drain Start"=w808, "Drain Stop"=w807, "Drain Step"=w806, "Drain Compliance"=w823, "Range mode"=w787, "Range"=w786) -> (w791:T7)
        n211 = call "4155C Output.vi"("VISA resource name in"=w793, "Gate"=w790, "Drain"=w791, "Timings"=w821, "error in (no error)"=w794, "SMU4"=w781, "sweep mode"=w814, "Panel controls"=w780) -> ("VD"=w778:dbl[], "Outparams"=w785:T9, "VISA Resource Name out"=w820:refnum<visa-resource-name>, "IS"=w745:dbl[], "ID"=w747:dbl[], "IG"=w744:dbl[], "error out"=w767:errorcluster, "SMU4"=w782:dbl[])  [unwired: 12 in]
        n212 = Unbundle By Name(w785) -> ("V2 Step"=w784:dbl, "V2 Start"=w783:dbl, "Number of points"=w714:i32)
        n213 = Absolute Value(x=w745) -> (abs(x)=w730:dbl[])
        n214 = Absolute Value(x=w747) -> (abs(x)=w746:dbl[])
        n215 = Absolute Value(x=w744) -> (abs(x)=w733:dbl[])
        n216 = Array Size(array=w746) -> (size(s)=w754:i32)
        n217 = Divide(x=w754, y=2) -> (x/y=w697:dbl)
        n218 = Subtract(x=w697, y=1) -> (x-y=w696:dbl)
        n219 = Array Max & Min(array=w730) -> (max value=w737:dbl, min value=w738:dbl)  [unwired: 2 out]
        n220 = Array Max & Min(array=w746) -> (max value=w776:dbl, min value=w743:dbl)  [unwired: 2 out]
        n221 = Array Max & Min(array=w733) -> (max value=w742:dbl, min value=w741:dbl)  [unwired: 2 out]
        n222 = call "4155C Split array.vi"("Number of VAR2 steps"=w714, "Y2 data in"=w747, "X data in"=w778, "Y1 data in"=w745, "Y3 data in"=w744, "error in (no error)"=w767) -> ("Array of clusters"=w769:cluster{"Y data in":dbl[], "X data in":dbl[]}[], "error out"=w702:errorcluster)  [unwired: 1 in]
        n223 = Index Array(array=w730, index=w696) -> (element=w721:dbl)
        n224 = Index Array(array=w730, index=0) -> (element=w722:dbl)
        n225 = Index Array(array=w746, index=w696) -> (element=w723:dbl)
        n226 = Index Array(array=w746, index=0) -> (element=w724:dbl)
        n227 = Index Array(array=w733, index=w696) -> (element=w726:dbl)
        n228 = Index Array(array=w733, index=0) -> (element=w725:dbl)
        n229 = local write "Ig max"(w742) -> ()
        n230 = local write "Ig min"(w741) -> ()
        n231 = local write "Is max"(w737) -> ()
        n232 = local write "Is min"(w738) -> ()
        n233 = local write "Id max"(w776) -> ()
        n234 = local write "Id min"(w743) -> ()
        n235 = local write "I vs Vd"(w769) -> ()
        n236 = Build Array (concatenate)(w736, w737) -> (w715:dbl[])
        n237 = Build Array (concatenate)(w735, w738) -> (w713:dbl[])
        n238 = local write "Is off"(w722) -> ()
        n239 = local write "Is on"(w721) -> ()
        n240 = Build Array (concatenate)(w777, w776) -> (w712:dbl[])
        n241 = Build Array (concatenate)(w764, w743) -> (w711:dbl[])
        n242 = Build Array (concatenate)(w740, w742) -> (w710:dbl[])
        n243 = Build Array (concatenate)(w739, w741) -> (w709:dbl[])
        n244 = Build Array (concatenate)(w728, w721) -> (w708:dbl[])
        n245 = Build Array (concatenate)(w727, w722) -> (w707:dbl[])
        n246 = Build Array (concatenate)(w750, w723) -> (w706:dbl[])
        n247 = Build Array (concatenate)(w751, w724) -> (w705:dbl[])
        n248 = Build Array (concatenate)(w732, w726) -> (w704:dbl[])
        n249 = Build Array (concatenate)(w731, w725) -> (w703:dbl[])
        n250 = local write "Ig off"(w725) -> ()
        n251 = local write "Ig on"(w726) -> ()
        n252 = local write "Id off"(w724) -> ()
        n253 = local write "Id on"(w723) -> ()
        n254 = call "4155C Split array.vi"("Number of VAR2 steps"=w714, "Y2 data in"=w706, "X data in"=w720, "Y1 data in"=w708, "Y3 data in"=w704, "error in (no error)"=w702) -> ("Array of clusters"=w718:cluster{"Y data in":dbl[], "X data in":dbl[]}[], "error out"=w701:errorcluster)  [unwired: 1 in]
        n255 = call "4155C Split array.vi"("Number of VAR2 steps"=w714, "Y2 data in"=w705, "X data in"=w720, "Y1 data in"=w707, "Y3 data in"=w703, "error in (no error)"=w701) -> ("Array of clusters"=w719:cluster{"Y data in":dbl[], "X data in":dbl[]}[], "error out"=w700:errorcluster)  [unwired: 1 in]
        n256 = call "4155C Split array.vi"("Number of VAR2 steps"=w714, "Y2 data in"=w712, "X data in"=w720, "Y1 data in"=w715, "Y3 data in"=w710, "error in (no error)"=w700) -> ("Array of clusters"=w768:cluster{"Y data in":dbl[], "X data in":dbl[]}[], "error out"=w699:errorcluster)  [unwired: 1 in]
        n257 = call "4155C Split array.vi"("Number of VAR2 steps"=w714, "Y2 data in"=w711, "X data in"=w720, "Y1 data in"=w713, "Y3 data in"=w709, "error in (no error)"=w699) -> ("Array of clusters"=w765:cluster{"Y data in":dbl[], "X data in":dbl[]}[], "error out"=w698:errorcluster)  [unwired: 1 in]
        n258 = Open/Create/Replace File(file path (use dialog)=w824, error in=w698, operation (0:open)=w779) -> (refnum out=w762:refnum<file>, error out=w760:errorcluster)  [unwired: 3 in, 1 out]
        n259 = call "4155C Make Big 2d array.vi"("1D Var1"=w778, "1d IS"=w745, "1d ID"=w747, "1d IG"=w744, "1d SMU4"=w782, "SMU4"=w781, "VAR2 START"=w783, "Number of VAR2 steps"=w714, "VAR2 STEP"=w784, "VAR1 Name"="Vd", "Decimal places in header"=i8 1, "VAR2 Name"="Vg") -> ("Header array"=w763:string[], "Data array"=w761:dbl[][])  [unwired: 14 in]
        n260 = local write "Imax vs time"(w768) -> ()
        n261 = local write "Imin vs time"(w765) -> ()
        n262 = local write "Ion vs time"(w718) -> ()
        n263 = local write "Ioff vs time"(w719) -> ()
        n264 = call "4155C Config Chart Colours.vi"("Numeric"=w714, "XY Graph 2"=w749) -> ()  [unwired: 6 in]
        n265 = call "4155C Config Chart Colours.vi"("Numeric"=w714, "XY Graph 2"=w748) -> ()  [unwired: 6 in]
        n266 = call "4155C Config Chart Colours.vi"("Numeric"=w714, "XY Graph 2"=w717) -> ()  [unwired: 6 in]
        n267 = call "4155C Config Chart Colours.vi"("Numeric"=w714, "XY Graph 2"=w716) -> ()  [unwired: 6 in]
        n268 = call "4155C Config Chart Colours.vi"("Numeric"=w714, "XY Graph 2"=w775) -> ()  [unwired: 6 in]
        n269 = call "4155C Write array to file.vi"("Byte Stream File Refnum"=w762, "Header"=w763, "Data Array"=w761, "error in (no error)"=w760) -> ("dup refnum"=w759:refnum<file>, "error out"=w758:errorcluster)  [unwired: 1 in]
        n270 = Close File(refnum=w759, error in=w758) -> (error out=w819:errorcluster)  [unwired: 1 out]
      }
      frame "output-fpp" {
        n271 = Number To Decimal String(number=w846) -> (decimal integer string=w900:string)  [unwired: 1 in]
        n272 = Bundle By Name(cluster=w876, "Emergency Stop"=w903) -> (w913:T2)
        n273 = Delete From Array(array=w891, index=0 ("Index")) -> (deleted portion=w889:string, array with subset deleted=w888:string[])  [unwired: 1 in]
        n274 = VISA Write(VISA resource name=w867, write buffer=":PAGE:CHAN:MODE SWE;" ("write buffer (\"\")"), error in (no error)=w864) -> (VISA resource name out=w866:refnum<visa-resource-name>, error out=w865:errorcluster)  [unwired: 1 out]
        n275 = Concatenate Strings(w899, "-outputfpp-" ("Substring"), w900, w845, ".txt" ("Substring")) -> (w902:string)
        n276 = case shown="\"d\", Default" w889 {
          tunnel: [w914 w915] -> w887
          frame "s" {
            w914 = u16 0 items=["Single", "Double"] ("sweep mode")
          }
          frame "d", Default {
            w915 = u16 1 items=["Single", "Double"] ("sweep mode")
          }
        }
        n277 = Fract/Exp String To Number(string=w888) -> (number=w870:dbl[])  [unwired: 3 in, 1 out]
        n278 = String To Path(string=w902) -> (path=w898:path)
        n279 = Index Array(array=w870, index #1=0 ("Index")) -> (element #1=w886:dbl, element #2=w885:dbl, element #3=w884:dbl)  [unwired: 2 in]
        n280 = Delete From Array(array=w870, length=3 ("Length"), index=0 ("Index")) -> (array with subset deleted=w869:dbl[])  [unwired: 1 out]
        n281 = Bundle By Name(cluster=w878, "Gate Start"=w886, "Gate Stop"=w885, "Gate Step (linear only)"=w884, "Gate Compliance"=w896, "Range mode"=w862, "Range"=w861) -> (w912:T6)
        n282 = Index Array(array=w869, index #1=0 ("Index")) -> (element #1=w881:dbl, element #2=w880:dbl, element #3=w879:dbl)  [unwired: 2 in]
        n283 = call <vilib>:"compatOverwrite.vi"("overwrite (F)"=TRUE) -> ("overwrite?"=w850:T8)
        n284 = Bundle By Name(cluster=w877, "Drain Start"=w881, "Drain Stop"=w880, "Drain Step"=w879, "Drain Compliance"=w897, "Range mode"=w860, "Range"=w863) -> (w911:T7)
        n285 = call "4155C Output-FPP.vi"("VISA resource name in"=w866, "Gate"=w912, "Drain"=w911, "Timings"=w895, "error in (no error)"=w865, "sweep mode"=w887, "Panel controls"=w913) -> ("VD"=w855:dbl[], "Outparams"=w858:T9, "VISA Resource Name out"=w893:refnum<visa-resource-name>, "Vprobe2"=w854:dbl[], "ID"=w853:dbl[], "IG"=w852:dbl[], "Vprobe1"=w851:dbl[], "error out"=w894:errorcluster)  [unwired: 13 in]
        n286 = Unbundle By Name(w858) -> ("V2 Step"=w859:dbl, "V2 Start"=w857:dbl, "Number of points"=w856:i32)
        n287 = Open/Create/Replace File(file path (use dialog)=w898, error in=w894, operation (0:open)=w850) -> (refnum out=w908:refnum<file>, error out=w909:errorcluster)  [unwired: 3 in, 1 out]
        n288 = call "4155C Make Big 2d array FPP.vi"("1D Var1"=w855, "1d ID"=w853, "1d Vp2"=w854, "1d IG"=w852, "1d Vp1"=w851, "VAR2 START"=w857, "Number of VAR2 steps"=w856, "VAR2 STEP"=w859, "VAR1 Name"="Vd", "Decimal places in header"=i8 1, "VAR2 Name"="Vg") -> ("Header array"=w904:string[], "Data array"=w905:dbl[][])  [unwired: 15 in]
        n289 = call "4155C Write array to file.vi"("Byte Stream File Refnum"=w908, "Header"=w904, "Data Array"=w905, "error in (no error)"=w909) -> ("dup refnum"=w906:refnum<file>, "error out"=w907:errorcluster)  [unwired: 1 in]
        n290 = Close File(refnum=w906, error in=w907) -> (error out=w892:errorcluster)  [unwired: 1 out]
      }
      frame "itime" {
        n291 = Delete From Array(array=w918, index=1) -> (deleted portion=w917:string)  [unwired: 1 in, 1 out]
        n292 = Delete From Array(array=w918, index=0 ("Index")) -> (deleted portion=w947:string)  [unwired: 1 in, 1 out]
        n293 = Fract/Exp String To Number(string=w917) -> (number=w916:dbl)  [unwired: 3 in, 1 out]
        n294 = case shown="\"l\"" w947 {
          tunnel: w946 -> [w952 w954 w958]
          tunnel: [w951 w953 w957] -> w939
          tunnel: w916 -> [w949 _ w956]
          frame "s" {
            w950 = u32 0 items=["short  ", "medium  ", "long  "] ("integration time 2")
            n295 = Bundle By Name(cluster=w952, "integration time"=w950, "Short/Long integration time"=w949) -> (w951:T5)
          }
          frame "m", Default {
            w955 = u32 1 items=["short  ", "medium  ", "long  "] ("integration time 2")
            n296 = Bundle By Name(cluster=w954, "integration time"=w955) -> (w953:T5)
          }
          frame "l" {
            w959 = u32 2 items=["short  ", "medium  ", "long  "] ("integration time 2")
            n297 = Bundle By Name(cluster=w958, "integration time"=w959, "Short/Long integration time"=w956) -> (w957:T5)
          }
        }
      }
      frame "pulsed" {
        n298 = Delete From Array(array=w988, index=0 ("Index")) -> (deleted portion=w989:string, array with subset deleted=w976:string[])  [unwired: 1 in]
        n299 = case shown="\"on\", Default" w989 {
          tunnel: w987 -> [w999 w1002]
          tunnel: [w998 w1001] -> w980
          tunnel: w976 -> [w996 _]
          frame "on", Default {
            w997 = u16 1 items=["Continuous", "Pulsed"] ("sweep method")
            n300 = Fract/Exp String To Number(string=w996) -> (number=w994:dbl[])  [unwired: 3 in, 1 out]
            n301 = Index Array(array=w994, index #1=0 ("Index")) -> (element #1=w993:dbl, element #2=w992:dbl, element #3=w991:dbl)  [unwired: 2 in]
            n302 = Bundle By Name(cluster=w999, "sweep method"=w997, "Pulse period"=w993, "Base voltage"=w992, "Pulse width"=w991) -> (w998:T5)
          }
          frame "off" {
            w1000 = u16 0 items=["Continuous", "Pulsed"] ("sweep method")
            n303 = Bundle By Name(cluster=w1002, "sweep method"=w1000) -> (w1001:T5)
          }
        }
      }
      frame "gaterangemode" {
        n304 = Delete From Array(array=w1029, index=0 ("Index")) -> (deleted portion=w1030:string)  [unwired: 1 in, 1 out]
        n305 = case shown="\"f\"" w1030 {
          tunnel: [w1032 w1033 w1034] -> w1019
          frame "a", Default {
            w1032 = u16 0 items=["Auto", "Limited", "Fixed"] ("Gate Range\nmode 2")
          }
          frame "f" {
            w1033 = u16 2 items=["Auto", "Limited", "Fixed"] ("Gate Range\nmode 2")
          }
          frame "l" {
            w1034 = u16 1 items=["Auto", "Limited", "Fixed"] ("Gate Range\nmode 2")
          }
        }
      }
      frame "gaterange" {
        (unwired) u8 11 items=["10fA  ", "100fA  ", "1nA  ", "10nA", "100nA", "1uA", "10uA", "100uA", "1mA", "10mA", "100mA", "1A"] ("Gate Range 2")
        n306 = Delete From Array(array=w1068, index=0 ("Index")) -> (deleted portion=w1058:string)  [unwired: 1 in, 1 out]
        n307 = Scan Value(string=w1058, format string="") -> (value=w1056:dbl)  [unwired: 1 in, 1 out]
        n308 = Logarithm Base 10(1:w1056) -> (0:w1055:dbl)
        n309 = Round To Nearest(number=w1055) -> (nearest integer value=w1054:dbl)
        n310 = Add(x=w1054, y=11.0) -> (x+y=w1052:dbl)
        n311 = To Unsigned Byte Integer(number=w1052) -> (unsigned 8bit integer=w1051:u8)
      }
      frame "drainrange" {
        (unwired) u8 11 items=["10fA  ", "100fA  ", "1nA  ", "10nA", "100nA", "1uA", "10uA", "100uA", "1mA", "10mA", "100mA", "1A"] ("Gate Range 2")
        n312 = Delete From Array(array=w1103, index=0 ("Index")) -> (deleted portion=w1094:string)  [unwired: 1 in, 1 out]
        n313 = Scan Value(string=w1094, format string="") -> (value=w1092:dbl)  [unwired: 1 in, 1 out]
        n314 = Logarithm Base 10(1:w1092) -> (0:w1091:dbl)
        n315 = Round To Nearest(number=w1091) -> (nearest integer value=w1090:dbl)
        n316 = Add(x=w1090, y=11.0) -> (x+y=w1088:dbl)
        n317 = To Unsigned Byte Integer(number=w1088) -> (unsigned 8bit integer=w1087:u8)
      }
      frame "drainrangemode" {
        n318 = Delete From Array(array=w1131, index=0 ("Index")) -> (deleted portion=w1132:string)  [unwired: 1 in, 1 out]
        n319 = case shown="\"f\"" w1132 {
          tunnel: [w1134 w1135 w1136] -> w1121
          frame "a", Default {
            w1134 = u16 0 items=["Auto", "Limited", "Fixed"] ("Gate Range\nmode 2")
          }
          frame "f" {
            w1135 = u16 2 items=["Auto", "Limited", "Fixed"] ("Gate Range\nmode 2")
          }
          frame "l" {
            w1136 = u16 1 items=["Auto", "Limited", "Fixed"] ("Gate Range\nmode 2")
          }
        }
      }
      frame "Error", Default {
      }
      frame "logfile" {
        n320 = Number To Decimal String(number=w1179) -> (decimal integer string=w1214:string)  [unwired: 1 in]
        n321 = Concatenate Strings(w1213, "logfile" ("Substring"), w1214, w1177, ".txt" ("Substring")) -> (w1211:string)
        n322 = String To Path(string=w1211) -> (path=w1184:path)
        n323 = Unbundle(w1210) -> ("integration time"=w1209:u32, "Short/Long integration time"=w1208:dbl, "hold time (sec)"=w1207:dbl, "delay time (sec)"=w1206:dbl, "Step Time (0 disables)"=w1205:dbl, "sweep method"=w1204:u16, "Pulse period"=w1203:dbl, "Base voltage"=w1202:dbl, "Pulse width"=w1201:dbl)
        n324 = Build Array(w1209, w1208, w1207, w1206, w1205, w1204, w1203, w1202, w1201, w1195, w1196, w1197, w1198, w1199, w1200) -> (w1188:dbl[])
        n325 = Insert Into Array(array=dbl[][] [] ("Input Array"), new element=w1188) -> (w1187:dbl[][])  [unwired: 2 in]
        n326 = call <vilib>:"compatOverwrite.vi"("overwrite (F)"=TRUE) -> ("overwrite?"=w1182:T8)
        n327 = Open/Create/Replace File(file path (use dialog)=w1184, error in=w1186, operation (0:open)=w1182) -> (refnum out=w1192:refnum<file>, error out=w1191:errorcluster)  [unwired: 3 in, 1 out]
        n328 = call "4155C Write array to file.vi"("Byte Stream File Refnum"=w1192, "Header"=string[] ["Int Time", "Short/Long Itime", "Hold time", "Delay time", "Step time", "Sweep method", "Pulse period", "Base Voltage", "Pulse width", "Drain compliance", "Gate compliance", "Gate range mode", "Gate range", "S/D range mode", "S/D range"], "Data Array"=w1187, "error in (no error)"=w1191) -> ("dup refnum"=w1194:refnum<file>, "error out"=w1193:errorcluster)  [unwired: 1 in]
        n329 = Close File(refnum=w1194, error in=w1193) -> (error out=w1185:errorcluster)  [unwired: 1 out]
      }
      frame "sample" {
        n330 = Number To Decimal String(number=w1232) -> (decimal integer string=w1280:string)  [unwired: 1 in]
        n331 = Fract/Exp String To Number(string=w1277) -> (number=w1238:dbl[])  [unwired: 3 in, 1 out]
        n332 = Concatenate Strings(w1255, "-sample-" ("Substring"), w1280, w1230, ".txt" ("Substring")) -> (w1278:string)
        n333 = Index Array(array=w1238, index=0 ("Index")) -> (element=w1275:dbl)
        n334 = String To Path(string=w1278) -> (path=w1259:path)
        n335 = Index Array(array=w1238, index=2 ("Index")) -> (element=w1271:dbl)
        n336 = Index Array(array=w1238, index=3 ("Index")) -> (element=w1240:dbl)
        n337 = Index Array(array=w1238, index=4 ("Index")) -> (element=w1237:dbl)
        n338 = call "4155C Config Sampling Measurements.vi"("Sampling interval"=w1237, "Sample time"=w1240, "Display on/off"=TRUE, "Timings"=w1246, "Num Points"=w1271, "error in (no error)"=w1282, "Drain Compliance"=w1281, "Gate Compliance"=w1256, "VISA session"=w1283) -> ("error out"=w1284:errorcluster, "dup VISA resource name"=w1285:refnum<visa-resource-name>)  [unwired: 1 in]
        n339 = Index Array(array=w1238, index=1 ("Index")) -> (element=w1272:dbl)
        n340 = call "4155C Take Sample.vi"("Emergency Stop"=w1252, "error in (no error)"=w1284, "Vd"=w1272, "Vg"=w1275, "VISA resource name in"=w1285) -> ("error out"=w1250:errorcluster, "Id"=w1287:dbl[], "Ig"=w1261:dbl[], "VISA Resource Name out"=w1248:refnum<visa-resource-name>, "Is"=w1286:dbl[], "Time"=w1265:dbl[])  [unwired: 1 in]
        n341 = Insert Into Array(array=dbl[][] [] ("Input Array"), new element=w1265) -> (w1264:dbl[][])  [unwired: 2 in]
        n342 = Insert Into Array(array=w1264, new element=w1261) -> (w1263:dbl[][])  [unwired: 2 in]
        n343 = Insert Into Array(array=w1263, new element=w1287) -> (w1262:dbl[][])  [unwired: 2 in]
        n344 = VISA Write(VISA resource name=w1248, write buffer=":DISP ON" ("write buffer (\"\")"), error in (no error)=w1250) -> (VISA resource name out=w1247:refnum<visa-resource-name>, error out=w1249:errorcluster)  [unwired: 1 out]
        n345 = Insert Into Array(array=w1262, new element=w1286) -> (w1254:dbl[][])  [unwired: 2 in]
        n346 = Transpose 2D Array(2D array=w1254) -> (transposed array=w1253:dbl[][])
        n347 = call <vilib>:"compatOverwrite.vi"("overwrite (F)"=TRUE) -> ("overwrite?"=w1235:T8)
        n348 = Open/Create/Replace File(file path (use dialog)=w1259, error in=w1249, operation (0:open)=w1235) -> (refnum out=w1268:refnum<file>, error out=w1267:errorcluster)  [unwired: 3 in, 1 out]
        n349 = call "4155C Write array to file.vi"("Byte Stream File Refnum"=w1268, "Header"=string[] ["Time /s", "Ig /A", "Id /A", "Is /A"], "Data Array"=w1253, "error in (no error)"=w1267) -> ("dup refnum"=w1270:refnum<file>, "error out"=w1269:errorcluster)  [unwired: 1 in]
        n350 = Close File(refnum=w1270, error in=w1269) -> (error out=w1257:errorcluster)  [unwired: 1 out]
      }
      frame "samplei" {
        n351 = Number To Decimal String(number=w1304) -> (decimal integer string=w1355:string)  [unwired: 1 in]
        n352 = Concatenate Strings(w1334, "-samplei-" ("Substring"), w1355, w1303, ".txt" ("Substring")) -> (w1353:string)
        n353 = Fract/Exp String To Number(string=w1352) -> (number=w1319:dbl[])  [unwired: 3 in, 1 out]
        n354 = String To Path(string=w1353) -> (path=w1337:path)
        n355 = Index Array(array=w1319, index=4 ("Index")) -> (element=w1313:dbl)
        n356 = Index Array(array=w1319, index=3 ("Index")) -> (element=w1314:dbl)
        n357 = Index Array(array=w1319, index=1 ("Index")) -> (element=w1316:dbl)
        n358 = Index Array(array=w1319, index=0 ("Index")) -> (element=w1317:dbl)
        n359 = Index Array(array=w1319, index=2 ("Index")) -> (element=w1315:dbl)
        n360 = call "4155C Config SamplingI Measurements.vi"("Sample time"=w1315, "Display on/off"=TRUE, "Timings"=w1326, "Num Points"=w1316, "error in (no error)"=w1357, "Sampling interval"=w1314, "VISA session"=w1358) -> ("error out"=w1359:errorcluster, "dup VISA resource name"=w1360:refnum<visa-resource-name>)  [unwired: 3 in]
        n361 = call "4155C Take SampleI.vi"("Emergency Stop"=w1331, "error in (no error)"=w1359, "Idg 2"=w1317, "Vdg compliance 2"=w1313, "VISA resource name in"=w1360) -> ("error out"=w1329:errorcluster, "Idg"=w1362:dbl[], "Vdg"=w1339:dbl[], "VISA Resource Name out"=w1327:refnum<visa-resource-name>, "Is"=w1361:dbl[], "Time"=w1343:dbl[])  [unwired: 1 in]
        n362 = Insert Into Array(array=dbl[][] [] ("Input Array"), new element=w1343) -> (w1342:dbl[][])  [unwired: 2 in]
        n363 = Insert Into Array(array=w1342, new element=w1339) -> (w1341:dbl[][])  [unwired: 2 in]
        n364 = Insert Into Array(array=w1341, new element=w1362) -> (w1340:dbl[][])  [unwired: 2 in]
        n365 = VISA Write(VISA resource name=w1327, write buffer=":DISP ON" ("write buffer (\"\")"), error in (no error)=w1329) -> (VISA resource name out=w1312:refnum<visa-resource-name>, error out=w1328:errorcluster)  [unwired: 1 out]
        n366 = Insert Into Array(array=w1340, new element=w1361) -> (w1333:dbl[][])  [unwired: 2 in]
        n367 = call <vilib>:"compatOverwrite.vi"("overwrite (F)"=TRUE) -> ("overwrite?"=w1307:T8)
        n368 = Open/Create/Replace File(file path (use dialog)=w1337, error in=w1328, operation (0:open)=w1307) -> (refnum out=w1346:refnum<file>, error out=w1345:errorcluster)  [unwired: 3 in, 1 out]
        n369 = Transpose 2D Array(2D array=w1333) -> (transposed array=w1332:dbl[][])
        n370 = call "4155C Write array to file.vi"("Byte Stream File Refnum"=w1346, "Header"=string[] ["Time /s", "Vdg /V", "Idg /A", "Is /A"], "Data Array"=w1332, "error in (no error)"=w1345) -> ("dup refnum"=w1348:refnum<file>, "error out"=w1347:errorcluster)  [unwired: 1 in]
        n371 = Close File(refnum=w1348, error in=w1347) -> (error out=w1310:errorcluster)  [unwired: 1 out]
        n372 = VISA Write(VISA resource name=w1312, write buffer=";:PAGE:SCON:STAN OFF;:PAGE:CHAN:VSU2:DIS;" ("write buffer (\"\")"), error in (no error)=w1310) -> (VISA resource name out=w1308:refnum<visa-resource-name>, error out=w1309:errorcluster)  [unwired: 1 out]
      }
      frame "#" {
        n373 = VISA Write(VISA resource name=w1383, write buffer=":DISP ON" ("write buffer (\"\")"), error in (no error)=w1382) -> (VISA resource name out=w1381:refnum<visa-resource-name>, error out=w1380:errorcluster)  [unwired: 1 out]
      }
      frame "stressV" {
        n374 = Number To Decimal String(number=w1407) -> (decimal integer string=w1448:string)  [unwired: 1 in]
        n375 = Concatenate Strings(w1432, "-stressV-" ("Substring"), w1448, w1406, ".txt" ("Substring")) -> (w1446:string)
        n376 = Fract/Exp String To Number(string=w1445) -> (number=w1418:dbl[])  [unwired: 3 in, 1 out]
        n377 = String To Path(string=w1446) -> (path=w1436:path)
        n378 = Index Array(array=w1418, index=3 ("Index")) -> (element=w1415:dbl)
        n379 = Index Array(array=w1418, index=1 ("Index")) -> (element=w1413:dbl)
        n380 = Index Array(array=w1418, index=0 ("Index")) -> (element=w1412:dbl)
        n381 = Index Array(array=w1418, index=4 ("Index")) -> (element=w1417:dbl)
        n382 = Index Array(array=w1418, index=2 ("Index")) -> (element=w1414:dbl)
        n383 = call "4155C Config V Stress.vi"("VISA session"=w1451, "ID compliance"=w1415, "VD"=w1413, "VG"=w1412, "IG compliance"=w1414, "error in (no error)"=w1450, "Display on/off"=TRUE) -> ("dup VISA resource name"=w1453:refnum<visa-resource-name>, "error out"=w1452:errorcluster)
        n384 = call "4155C Apply Stress.vi"("error in (no error)"=w1452, "Duration"=w1417, "Emergency Stop"=w1431, "VISA resource name in"=w1453) -> ("error out"=w1429:errorcluster, "VISA Resource Name out"=w1427:refnum<visa-resource-name>)
        n385 = VISA Write(VISA resource name=w1427, write buffer=":DISP ON" ("write buffer (\"\")"), error in (no error)=w1429) -> (VISA resource name out=w1426:refnum<visa-resource-name>, error out=w1428:errorcluster)  [unwired: 1 out]
        n386 = call <vilib>:"compatOverwrite.vi"("overwrite (F)"=TRUE) -> ("overwrite?"=w1411:T8)
        n387 = Open/Create/Replace File(file path (use dialog)=w1436, error in=w1428, operation (0:open)=w1411) -> (refnum out=w1439:refnum<file>, error out=w1438:errorcluster)  [unwired: 3 in, 1 out]
        n388 = call "4155C Write array to file.vi"("Byte Stream File Refnum"=w1439, "Header"=string[] ["V stress completed successfully", ""], "error in (no error)"=w1438) -> ("dup refnum"=w1441:refnum<file>, "error out"=w1440:errorcluster)  [unwired: 2 in]
        n389 = Close File(refnum=w1441, error in=w1440) -> (error out=w1434:errorcluster)  [unwired: 1 out]
      }
      frame "stressI" {
        n390 = Number To Decimal String(number=w1469) -> (decimal integer string=w1506:string)  [unwired: 1 in]
        n391 = Concatenate Strings(w1490, "-stressI-" ("Substring"), w1506, w1468, ".txt" ("Substring")) -> (w1504:string)
        n392 = Fract/Exp String To Number(string=w1503) -> (number=w1478:dbl[])  [unwired: 3 in, 1 out]
        n393 = Index Array(array=w1478, index=1 ("Index")) -> (element=w1474:dbl)
        n394 = Index Array(array=w1478, index=0 ("Index")) -> (element=w1475:dbl)
        n395 = call "4155C Config I Stress.vi"("VISA session"=w1509, "IDG"=w1475, "VDG compliance"=w1474, "error in (no error)"=w1508, "Display on/off"=TRUE) -> ("dup VISA resource name"=w1511:refnum<visa-resource-name>, "error out"=w1510:errorcluster)
        n396 = Index Array(array=w1478, index=2 ("Index")) -> (element=w1476:dbl)
        n397 = String To Path(string=w1504) -> (path=w1494:path)
        n398 = call "4155C Apply Stress.vi"("error in (no error)"=w1510, "Duration"=w1476, "Emergency Stop"=w1489, "VISA resource name in"=w1511) -> ("error out"=w1487:errorcluster, "VISA Resource Name out"=w1485:refnum<visa-resource-name>)
        n399 = VISA Write(VISA resource name=w1485, write buffer=":DISP ON" ("write buffer (\"\")"), error in (no error)=w1487) -> (VISA resource name out=w1484:refnum<visa-resource-name>, error out=w1486:errorcluster)  [unwired: 1 out]
        n400 = call <vilib>:"compatOverwrite.vi"("overwrite (F)"=TRUE) -> ("overwrite?"=w1473:T8)
        n401 = Open/Create/Replace File(file path (use dialog)=w1494, error in=w1486, operation (0:open)=w1473) -> (refnum out=w1497:refnum<file>, error out=w1496:errorcluster)  [unwired: 3 in, 1 out]
        n402 = call "4155C Write array to file.vi"("Byte Stream File Refnum"=w1497, "Header"=string[] ["I stress completed successfully", ""], "error in (no error)"=w1496) -> ("dup refnum"=w1499:refnum<file>, "error out"=w1498:errorcluster)  [unwired: 2 in]
        n403 = Close File(refnum=w1499, error in=w1498) -> (error out=w1492:errorcluster)  [unwired: 1 out]
      }
      frame "vsu2pulse" {
        n404 = Number To Decimal String(number=w1527) -> (decimal integer string=w1562:string)  [unwired: 1 in]
        n405 = Concatenate Strings(w1547, "-vsu2-" ("Substring"), w1562, w1526, ".txt" ("Substring")) -> (w1560:string)
        n406 = Fract/Exp String To Number(string=w1559) -> (number=w1535:dbl[])  [unwired: 3 in, 1 out]
        n407 = String To Path(string=w1560) -> (path=w1551:path)
        n408 = Index Array(array=w1535, index=1 ("Index")) -> (element=w1534:dbl)
        n409 = Index Array(array=w1535, index=0 ("Index")) -> (element=w1532:dbl)
        n410 = call "4155C Config VSU2 Stress.vi"("error in (no error)"=w1564, "VSU2"=w1532, "Display on/off"=TRUE, "VISA session"=w1565) -> ("error out"=w1566:errorcluster, "dup VISA resource name"=w1567:refnum<visa-resource-name>)
        n411 = call "4155C Apply Stress.vi"("error in (no error)"=w1566, "Duration"=w1534, "Emergency Stop"=w1546, "VISA resource name in"=w1567) -> ("error out"=w1544:errorcluster, "VISA Resource Name out"=w1542:refnum<visa-resource-name>)
        n412 = VISA Write(VISA resource name=w1542, write buffer=":DISP ON" ("write buffer (\"\")"), error in (no error)=w1544) -> (VISA resource name out=w1541:refnum<visa-resource-name>, error out=w1543:errorcluster)  [unwired: 1 out]
        n413 = call <vilib>:"compatOverwrite.vi"("overwrite (F)"=TRUE) -> ("overwrite?"=w1531:T8)
        n414 = Open/Create/Replace File(file path (use dialog)=w1551, error in=w1543, operation (0:open)=w1531) -> (refnum out=w1554:refnum<file>, error out=w1553:errorcluster)  [unwired: 3 in, 1 out]
        n415 = call "4155C Write array to file.vi"("Byte Stream File Refnum"=w1554, "Header"=string[] ["VSU2 pulse completed successfully", ""], "error in (no error)"=w1553) -> ("dup refnum"=w1556:refnum<file>, "error out"=w1555:errorcluster)  [unwired: 2 in]
        n416 = Close File(refnum=w1556, error in=w1555) -> (error out=w1549:errorcluster)  [unwired: 1 out]
      }
      frame "sample-fpp" {
        w1594 = string[] ["Time /s", "Id VgVd /A", "Ig VgVd /A", "Vp1 VgVd /V", "Vp2 VgVd /V"] ("Header")
        w1598 = "%d" ("format string")
        n417 = Number To Decimal String(number=w1583) -> (decimal integer string=w1646:string)  [unwired: 1 in]
        n418 = Fract/Exp String To Number(string=w1643) -> (number=w1631:dbl[])  [unwired: 3 in, 1 out]
        n419 = Concatenate Strings(w1637, "-samplefpp-" ("Substring"), w1646, w1582, ".txt" ("Substring")) -> (w1644:string)
        n420 = String To Path(string=w1644) -> (path=w1606:path)
        n421 = Index Array(array=w1631, index=0 ("Index")) -> (element=w1592:dbl)
        n422 = Index Array(array=w1631, index=1 ("Index")) -> (element=w1591:dbl)
        n423 = Index Array(array=w1631, index=2 ("Index")) -> (element=w1639:dbl)
        n424 = Index Array(array=w1631, index=3 ("Index")) -> (element=w1629:dbl)
        n425 = call "4155C Config Sampling Measurements FPP.vi"("VISA session"=w1649, "Num Points"=w1639, "Vg"=w1592, "Display on/off"=TRUE, "Gate Compliance"=w1638, "Drain Compliance"=w1647, "Standby"="Standby", "error in (no error)"=w1648, "Timings"=w1636, "Vd"=w1591, "Sample time"=w1629) -> ("dup VISA resource name"=w1608:refnum<visa-resource-name>, "error out"=w1607:errorcluster)  [unwired: 3 in]
        n426 = Number To Decimal String(number=w1592) -> (decimal integer string=w1618:string)  [unwired: 1 in]
        n427 = call "4155C Take Sample FPP.vi"("VISA resource name in"=w1608, "error in (no error)"=w1607, "Emergency Stop"=w1609) -> ("Time"=w1613:dbl[], "Vp1"=w1623:dbl[], "VISA Resource Name out"=w1589:refnum<visa-resource-name>, "Ig"=w1611:dbl[], "Id"=w1612:dbl[], "Vp2"=w1621:dbl[], "error out"=w1610:errorcluster)  [unwired: 10 in]
        n428 = Insert Into Array(array=dbl[][] [] ("Input Array"), new element=w1613) -> (w1627:dbl[][])  [unwired: 2 in]
        n429 = Number To Decimal String(number=w1591) -> (decimal integer string=w1616:string)  [unwired: 1 in]
        n430 = Insert Into Array(array=w1627, new element=w1612) -> (w1626:dbl[][])  [unwired: 2 in]
        n431 = Concatenate Strings("(Vg = " ("Substring"), w1618, "V, Vd = " ("Substring"), w1616, "V)" ("Substring")) -> (w1614:string)
        n432 = Insert Into Array(array=w1626, new element=w1611) -> (w1625:dbl[][])  [unwired: 2 in]
        n433 = Insert Into Array(array=w1625, new element=w1623) -> (w1622:dbl[][])  [unwired: 2 in]
        n434 = Insert Into Array(array=w1622, new element=w1621) -> (w1590:dbl[][])  [unwired: 2 in]
        n435 = Transpose 2D Array(2D array=w1590) -> (transposed array=w1620:dbl[][])
        n436 = call <vilib>:"compatOverwrite.vi"("overwrite (F)"=TRUE) -> ("overwrite?"=w1587:T8)
        n437 = Open/Create/Replace File(file path (use dialog)=w1606, error in=w1610, operation (0:open)=w1587) -> (refnum out=w1603:refnum<file>, error out=w1604:errorcluster)  [unwired: 3 in, 1 out]
        n438 = Array To Spreadsheet String(array=w1594, 3:w1598) -> (spreadsheet string=w1600:string)  [unwired: 1 in]
        n439 = Search and Replace String(replace all?=TRUE ("replace all? (F)"), input string=w1600, search string="VgVd", replace string=w1614) -> (result string=w1596:string)  [unwired: 4 in, 3 out]
        n440 = Spreadsheet String To Array(format string=w1598, spreadsheet string=w1596, array type (2D Dbl)=w1594) -> (array=w1595:string[])  [unwired: 1 in]
        n441 = call "4155C Write array to file.vi"("Byte Stream File Refnum"=w1603, "Header"=w1595, "Data Array"=w1620, "error in (no error)"=w1604) -> ("dup refnum"=w1601:refnum<file>, "error out"=w1602:errorcluster)  [unwired: 1 in]
        n442 = Close File(refnum=w1601, error in=w1602) -> (error out=w1588:errorcluster)  [unwired: 1 out]
      }
      frame "resample-fpp" {
        w1678 = string[] ["Time /s", "Id VgVd /A", "Ig VgVd /A", "Vp1 VgVd /V", "Vp2 VgVd /V"] ("Header")
        w1682 = "%d" ("format string")
        n443 = Number To Decimal String(number=w1664) -> (decimal integer string=w1722:string)  [unwired: 1 in]
        n444 = Fract/Exp String To Number(string=w1719) -> (number=w1671:dbl[])  [unwired: 3 in, 1 out]
        n445 = Concatenate Strings(w1715, "-resamplefpp-" ("Substring"), w1722, w1665, ".txt" ("Substring")) -> (w1720:string)
        n446 = String To Path(string=w1720) -> (path=w1690:path)
        n447 = Index Array(array=w1671, index=0 ("Index")) -> (element=w1677:dbl)
        n448 = Index Array(array=w1671, index=1 ("Index")) -> (element=w1676:dbl)
        n449 = Number To Decimal String(number=w1677) -> (decimal integer string=w1700:string)  [unwired: 1 in]
        n450 = call "4155C Take Sample FPP.vi"("VISA resource name in"=w1673, "error in (no error)"=w1672, "Emergency Stop"=w1691) -> ("Time"=w1695:dbl[], "Vp1"=w1705:dbl[], "VISA Resource Name out"=w1675:refnum<visa-resource-name>, "Ig"=w1693:dbl[], "Id"=w1694:dbl[], "Vp2"=w1703:dbl[], "error out"=w1692:errorcluster)  [unwired: 10 in]
        n451 = Insert Into Array(array=dbl[][] [] ("Input Array"), new element=w1695) -> (w1709:dbl[][])  [unwired: 2 in]
        n452 = Number To Decimal String(number=w1676) -> (decimal integer string=w1698:string)  [unwired: 1 in]
        n453 = Insert Into Array(array=w1709, new element=w1694) -> (w1708:dbl[][])  [unwired: 2 in]
        n454 = Concatenate Strings("(Vg = " ("Substring"), w1700, "V, Vd = " ("Substring"), w1698, "V)" ("Substring")) -> (w1696:string)
        n455 = Insert Into Array(array=w1708, new element=w1693) -> (w1707:dbl[][])  [unwired: 2 in]
        n456 = Insert Into Array(array=w1707, new element=w1705) -> (w1704:dbl[][])  [unwired: 2 in]
        n457 = Insert Into Array(array=w1704, new element=w1703) -> (w1670:dbl[][])  [unwired: 2 in]
        n458 = call <vilib>:"compatOverwrite.vi"("overwrite (F)"=TRUE) -> ("overwrite?"=w1669:T8)
        n459 = Open/Create/Replace File(file path (use dialog)=w1690, error in=w1692, operation (0:open)=w1669) -> (refnum out=w1687:refnum<file>, error out=w1688:errorcluster)  [unwired: 3 in, 1 out]
        n460 = Array To Spreadsheet String(array=w1678, 3:w1682) -> (spreadsheet string=w1684:string)  [unwired: 1 in]
        n461 = Transpose 2D Array(2D array=w1670) -> (transposed array=w1702:dbl[][])
        n462 = Search and Replace String(replace all?=TRUE ("replace all? (F)"), input string=w1684, search string="VgVd", replace string=w1696) -> (result string=w1680:string)  [unwired: 4 in, 3 out]
        n463 = Spreadsheet String To Array(format string=w1682, spreadsheet string=w1680, array type (2D Dbl)=w1678) -> (array=w1679:string[])  [unwired: 1 in]
        n464 = call "4155C Write array to file.vi"("Byte Stream File Refnum"=w1687, "Header"=w1679, "Data Array"=w1702, "error in (no error)"=w1688) -> ("dup refnum"=w1685:refnum<file>, "error out"=w1686:errorcluster)  [unwired: 1 in]
        n465 = Close File(refnum=w1685, error in=w1686) -> (error out=w1674:errorcluster)  [unwired: 1 out]
      }
      frame "serial" {
        n466 = local read "Termination char\n(0xA = '\\n' = LF)\n(0xD = '\\r' = CR)"() -> (w1745:u8)
        n467 = local read "Enable Termination\nChar (T)"() -> (w1746:bool)
        n468 = Index Array(array=w1753, index=0 ("Index")) -> (element=w1752:string)
        n469 = local read "parity"() -> (w1736:u16)
        n470 = local read "Delay before read (ms)"() -> (w1747:u32)
        n471 = local read "byte count"() -> (w1744:u32)
        n472 = local read "Timeout (ms)"() -> (w1743:u32)
        n473 = local read "VISA resource name"() -> (w1740:refnum<visa-resource-name>)
        n474 = local read "baud rate"() -> (w1739:u32)
        n475 = local read "Serial End Mode for Reads"() -> (w1738:u16)
        n476 = local read "data bits"() -> (w1737:u16)
        n477 = local read "stop bits"() -> (w1742:u16)
        n478 = local read "flow control"() -> (w1741:u16)
        n479 = call "Serial write and read v0.5.vi"("Delay before read (ms)"=w1747, "Termination char\n(0xA = '\\n' = LF)\n(0xD = '\\r' = CR)"=w1745, "Enable Termination\nChar (T)"=w1746, "parity"=w1736, "stop bits"=w1742, "string to write"=w1752, "flow control"=w1741, "byte count"=w1744, "Serial Settings:Serial End Mode for Reads"=w1738, "Timeout (ms)"=w1743, "error in (no error)"=w1758, "VISA resource name"=w1740, "baud rate"=w1739, "data bits"=w1737) -> ("Serial port output"=w1748:string, "error out"=w1757:errorcluster)
        n480 = Build Array (concatenate)(w1748, w1749) -> (w1750:string[])
      }
    }
    n481 = Build Array(w113, w68, w78, w77, w76, w75, w74, w73, w72, w71, w70, w69, w67) -> (w137:dbl[][])
    n482 = Transpose 2D Array(2D array=w137) -> (transposed array=w136:dbl[][])
    n483 = Concatenate Strings(w65, "-Imax_Imin_Ion_Ioff_vs_time.txt" ("Suffix (Imax,Imin,Ion,Ioff)")) -> (w147:string)
    n484 = Build Array(w100, "Is max (A)" ("VAR2 Name"), "Is min (A)" ("VAR2 Name"), "Id max (A)" ("VAR2 Name"), "Id min (A)" ("VAR2 Name"), "Ig max (A)" ("VAR2 Name"), "Ig min (A)" ("VAR2 Name"), "Is on (A)" ("VAR2 Name"), "Is off (A)" ("VAR2 Name"), "Id on (A)" ("VAR2 Name"), "Id off (A)" ("VAR2 Name"), "Ig on (A)" ("VAR2 Name"), "Ig off (A)" ("VAR2 Name")) -> (w142:string[])
    n485 = Array To Spreadsheet String(array=w136, 3:"%e" ("format string")) -> (spreadsheet string=w140:string)  [unwired: 1 in]
    n486 = Array To Spreadsheet String(array=w142, 3:"" ("format string")) -> (spreadsheet string=w141:string)  [unwired: 1 in]
    n487 = String To Path(string=w147) -> (path=w146:path)
    n488 = Build Array(w141, w140) -> (w139:string[])
    n489 = Write to Text File(file (use dialog)=w146, text=w139, error in=w111) -> (refnum out=w148:refnum<file>, error out=w138:errorcluster)  [unwired: 1 in, 1 out]
    n490 = Close File(refnum=w148, error in=w138) -> (error out=w64:errorcluster)  [unwired: 1 out]
    n491 = Concatenate Strings(w65, "-serial_port_output.txt" ("Suffix (serial port log)")) -> (w117:string)
    n492 = String To Path(string=w117) -> (path=w116:path)
    n493 = Build Array(w100, "Serial port input" ("VAR2 Name"), "Serial port output: ") -> (w104:string[])
    n494 = Array To Spreadsheet String(array=w108, 3:"" ("format string")) -> (spreadsheet string=w101:string)  [unwired: 1 in]
    n495 = Array To Spreadsheet String(array=w104, 3:"" ("format string")) -> (spreadsheet string=w102:string)  [unwired: 1 in]
    n496 = Build Array(w102, w101) -> (w103:string[])
    n497 = Array To Spreadsheet String(array=w107, 3:"" ("format string")) -> (spreadsheet string=w122:string)  [unwired: 1 in]
    n498 = Write to Text File(file (use dialog)=w116, text=w103, error in=w64) -> (refnum out=w118:refnum<file>, error out=w119:errorcluster)  [unwired: 1 in, 1 out]
    n499 = Close File(refnum=w118, error in=w119) -> (error out=w62:errorcluster)  [unwired: 1 out]
    n500 = local write "Serial port data"(w122) -> ()
  }
  "error out" <- w24
  "Timings Indicator" <- w12
  "Is max" <- w6
  "Id max" <- w6
  "Ig max" <- w6
  "Imax vs time" <- w2
  "I vs Vg" <- w2
  "Imin vs time" <- w2
  "I vs Vd" <- w2
  "Serial port data" <- "" ("Serial port data")
  "Is min" <- w5
  "Id min" <- w5
  "Ig min" <- w5
  "Ion vs time" <- w2
  "Ioff vs time" <- w2
  "Is on" <- w4
  "Id on" <- w4
  "Ig on" <- w4
  "Is off" <- w3
  "Id off" <- w3
  "Ig off" <- w3
